vi "All-In-One_EIC-DIRC_DAQ_v2.vi"() -> ()   [LabVIEW 2024]
uses:
  C:/Users/hpDIRC/Desktop/eic_dirc_daq-LabVIEW_new/Thorlabs.MotionControl.Controls.dll
  Thorlabs.MotionControl.Controls.dll
  <vilib>/numeric/Random Number (Range) DBL.vi
  C:/Users/hpDIRC/Desktop/eic_dirc_daq-LabVIEW_new/Thorlabs.MotionControl.IntegratedStepperMotorsCLI.dll
  Thorlabs.MotionControl.IntegratedStepperMotorsCLI.dll
  C:/Users/hpDIRC/Desktop/eic_dirc_daq-LabVIEW_new/Thorlabs.MotionControl.Benchtop.StepperMotorCLI.dll
  Thorlabs.MotionControl.Benchtop.StepperMotorCLI.dll
  <instrlib>/Keithley 6517/Keithley 6517.lvlib
panel:
  in  "align-only":bool
  in  "run-BA":bool
  in  "run-IR":bool
  out "meter-mode":bool=TRUE
  in  "PDY start":dbl=105.8
  in  "PDX start":dbl=265.0
  out "run time (min)":dbl
  in  "align-only":bool
  out "alignment-counter":dbl=184.0 format="%#_13g"
  out "Optimized Location":dbl[](array[numeric])
  in  "Test Start Delay (s)":dbl=30.0
  out "Queue % Left":dbl format="%#_3g"
  out "next-state-cluster-const":T1={"next-state"="", "bypass-confirm"=FALSE, "PDX"=300.0, "PDY"=150.0, "BarX"=300.0, "BarY"=150.0, "BMA"=45.0, "PDA"=85.0, "bar-note"=0, "meas#"=0}
  in  "X start":dbl=262.0
  in  "X end":dbl=263.0
  in  "Y end":dbl=121.5 format="%#_13g"
  in  "X step size":dbl=0.2 format="%#_13g"
  in  "Y step size":dbl=0.2
  in  "Y start":dbl=120.5 format="%#_13g"
  in  "centered-diode-scan":bool
  out "keep-file":bool
  out "status":string
  out "queue-size":i32
  in  "save-loc":bool
  out "stored-pos":T2 caption="Location Stored"
  out "main-stage-refs":T3
  out "state-queue":T4(array[cluster])
  in  "PDA":dbl=184.0 format="%#_13g"
  in  "BMA":dbl=45.0 format="%#_13g"
  in  "BarY":dbl=30.0 format="%#_13g"
  in  "BarX":dbl=230.0 format="%#_13g"
  in  "PDY":dbl=124.0 format="%#_13g"
  in  "PDX":dbl=274.0 format="%#_13g"
  out "bypass-confirm":bool
  out "PD Values":cluster{"PD1":dbl, "PD2":dbl, "PD3":dbl}
  out "last-PD":dbl[](array[numeric])=[1.0, 1.0, 1.0]
  in  "move-bar":bool
  out "pd_angle":dbl
  out "brewster_angle":dbl
  out "meter-visa":refnum<visa-resource-name>
  out "loop-rate":u32
  out "meter-stat":bool caption="Log Status"
  out "file-stat":bool caption="Log Status"
  out "stage-stat":bool caption="Log Status"
  out "last-save-time":string caption="Time of Last Save:"
  out "pd_y_pos":dbl
  out "pd_x_pos":dbl
  out "bar_y_pos":dbl
  out "bar_x_pos":dbl
  in  "nSamples":dbl=50.0 caption="# Samples"
  out "Current Time:":string
  in  "save-data":bool
  in  "bar-note":u16(ring) items=["Pure Beam (PB)", "Internal Reflection (IR)", "Bulk Attenuation (BA)"]
  out "pd3_v":dbl caption="PD 3" format="%#.4g"
  out "pd2_v":dbl caption="PD 2" format="%#.4g"
  out "pd1_v":dbl caption="PD 1" format="%#.4g"
  out "meter-error":errorcluster
  out "log-error":errorcluster
  out "log-path":path caption="Path Data Will Save To:"
  out "start-msg":string
  out "stage-error":errorcluster
  in  "PD Angle":refnum<k24>(container)
  in  "Brewster":refnum<k24>(container)
  in  "PD Y":refnum<k24>(container)
  in  "PD X":refnum<k24>(container)
  in  "BAR Y":refnum<k24>(container)
  in  "stop":bool
  in  "BAR X":refnum<k24>(container)
  out "pd-plt":cluster{"[0]":dbl, "[1]":dbl, "[2]":dbl}(graph) caption="Measurement History"
  # "EXPERT DEBUGGING INFO"
  # "A"
  # "A"
  # "A"
  # "Work In Progress - please do not use"
  # "PD ONLY SCAN - CENTERED"
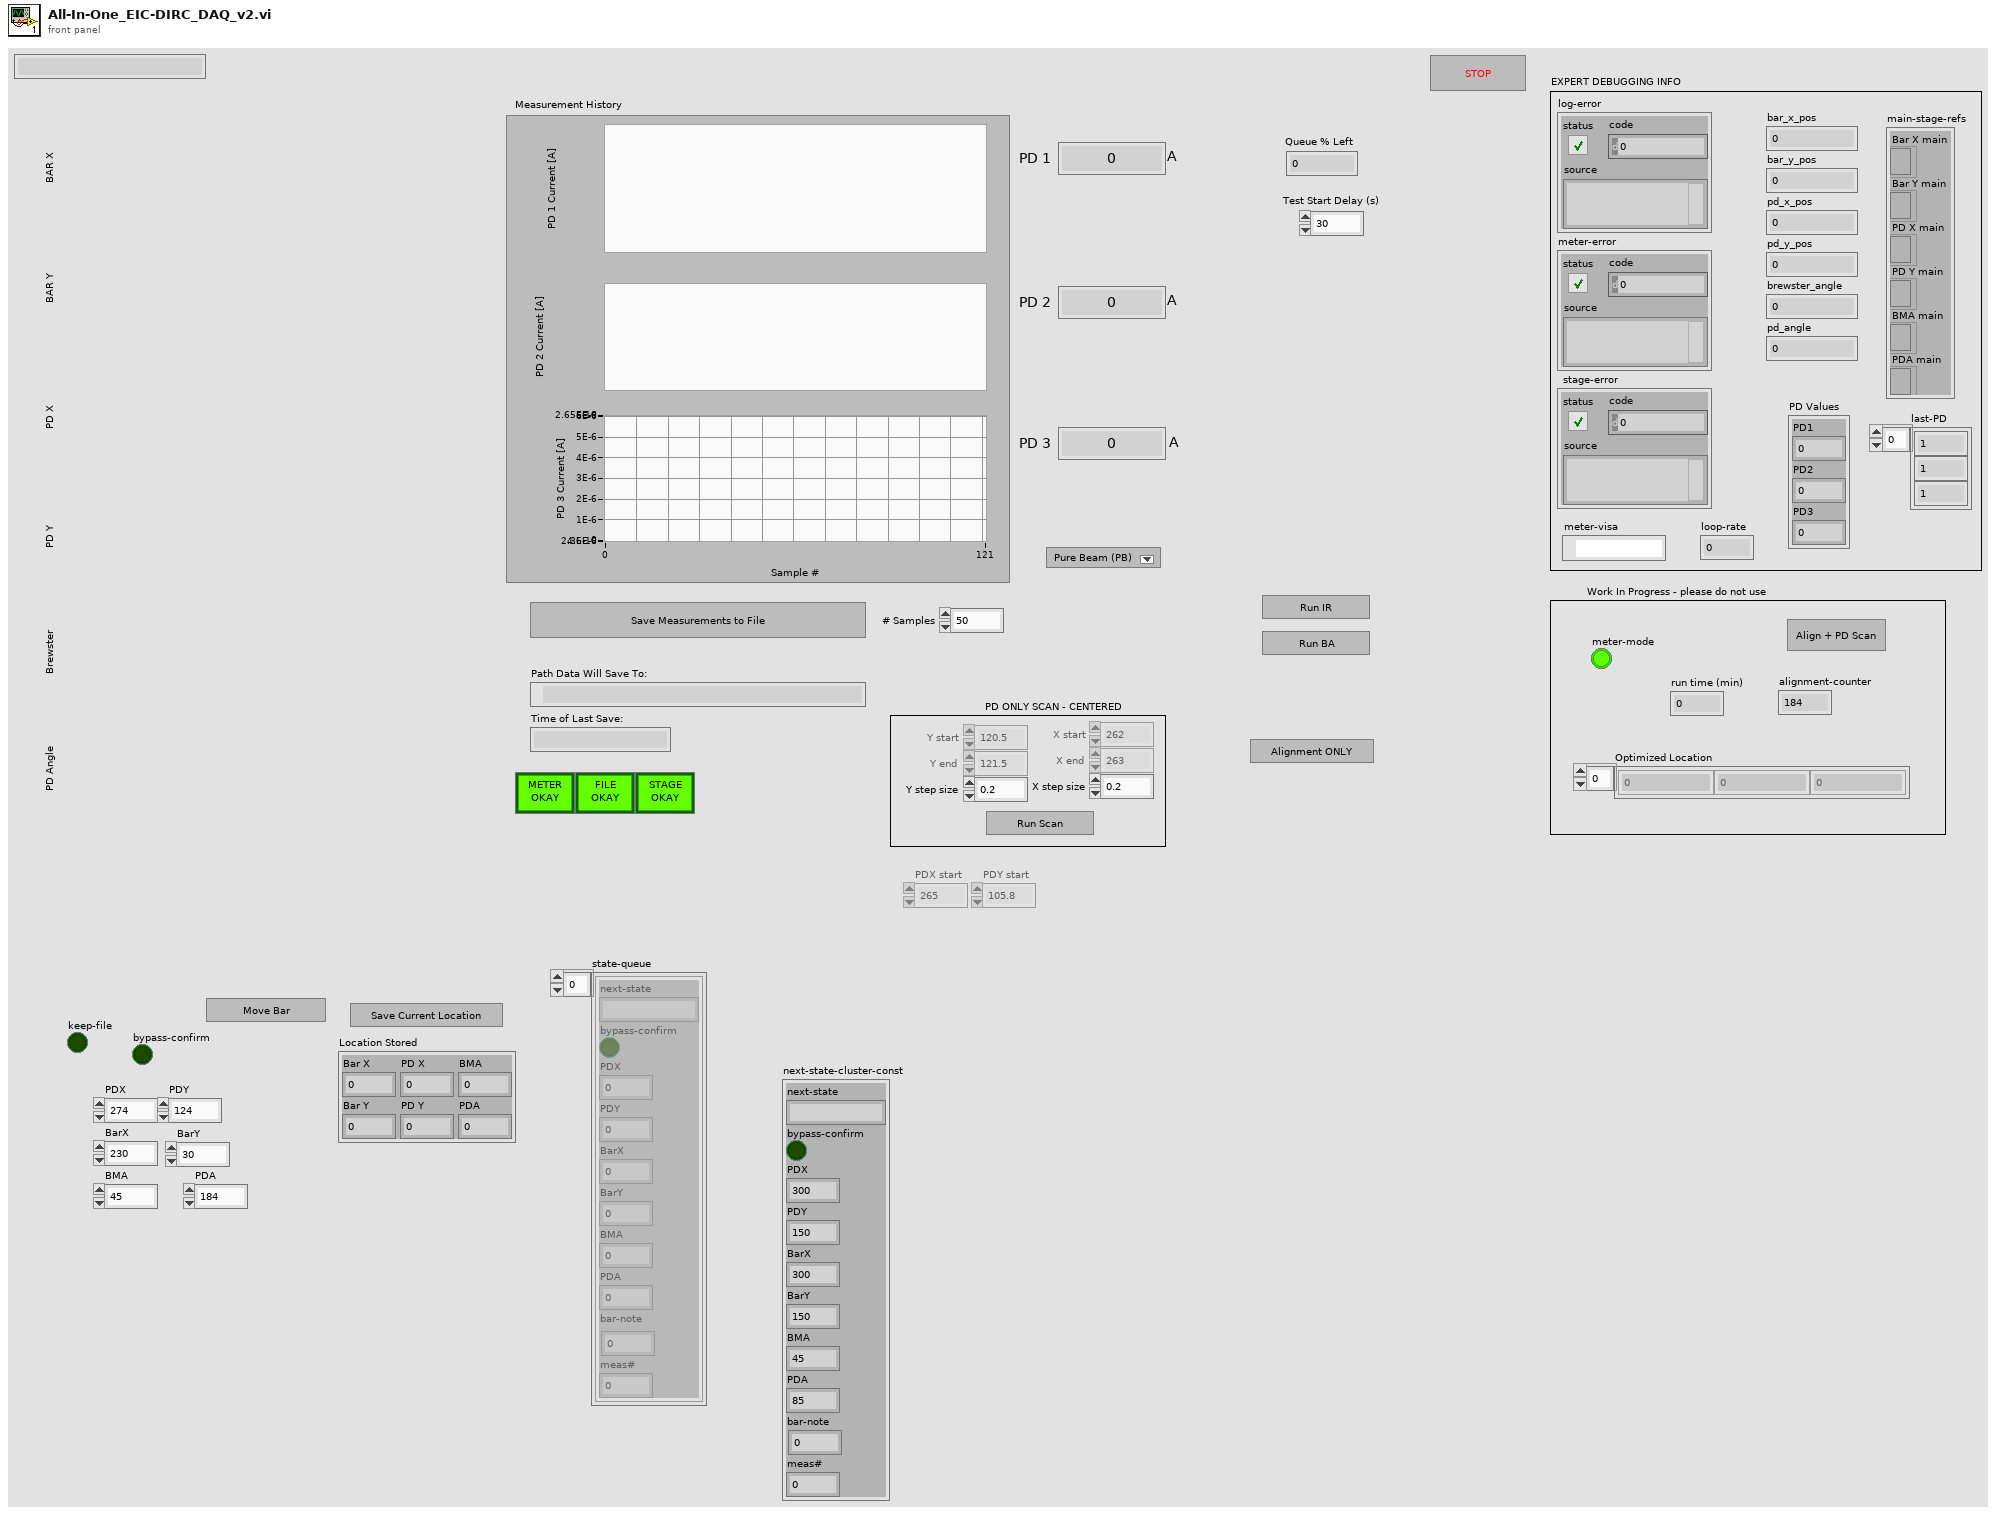
[diagram p1: front panel]
types:
  T1 = cluster{"next-state":string, "bypass-confirm":bool, "PDX":dbl, "PDY":dbl, "BarX":dbl, "BarY":dbl, "BMA":dbl, "PDA":dbl, "bar-note":u8, "meas#":u32}
  T2 = cluster{"Bar X":dbl, "Bar Y":dbl, "PD X":dbl, "PD Y":dbl, "BMA":dbl, "PDA":dbl}
  T3 = cluster{"Bar X main":refnum<k24>, "Bar Y main":refnum<k24>, "PD X main":refnum<k24>, "PD Y main":refnum<k24>, "BMA main":refnum<k24>, "PDA main":refnum<k24>}
  T4 = cluster{"next-state":string, "bypass-confirm":bool, "PDX":dbl, "PDY":dbl, "BarX":dbl, "BarY":dbl, "BMA":dbl, "PDA":dbl, "bar-note":u8, "meas#":u32}[]
  T5 = cluster{"Bar X":refnum<k24>, "Bar Y":refnum<k24>, "PD X":refnum<k24>, "PD Y":refnum<k24>, "Brewster":refnum<k24>, "PD Angle":refnum<k24>}
  T6 = enum16{"open", "replace", "create", "open or create", "replace or create", "replace or create with confirmation"}
  T7 = cluster{"alpha":dbl, "gamma":dbl, "rho":dbl, "sigma":dbl, "simplex L":dbl}
  T8 = cluster{"next-state":string, "mode-select":enum32{"IR", "Pure", "Bulk", "Bar Out", "stored-loc", "custom"}, "bypass-confirm":bool, "PDX":dbl, "PDY":dbl, "BarX":dbl, "BarY":dbl, "BMA":dbl, "PDA":dbl, "bar-note":bool}
  T9 = cluster{"error":bool, "code":i32, "source":string}
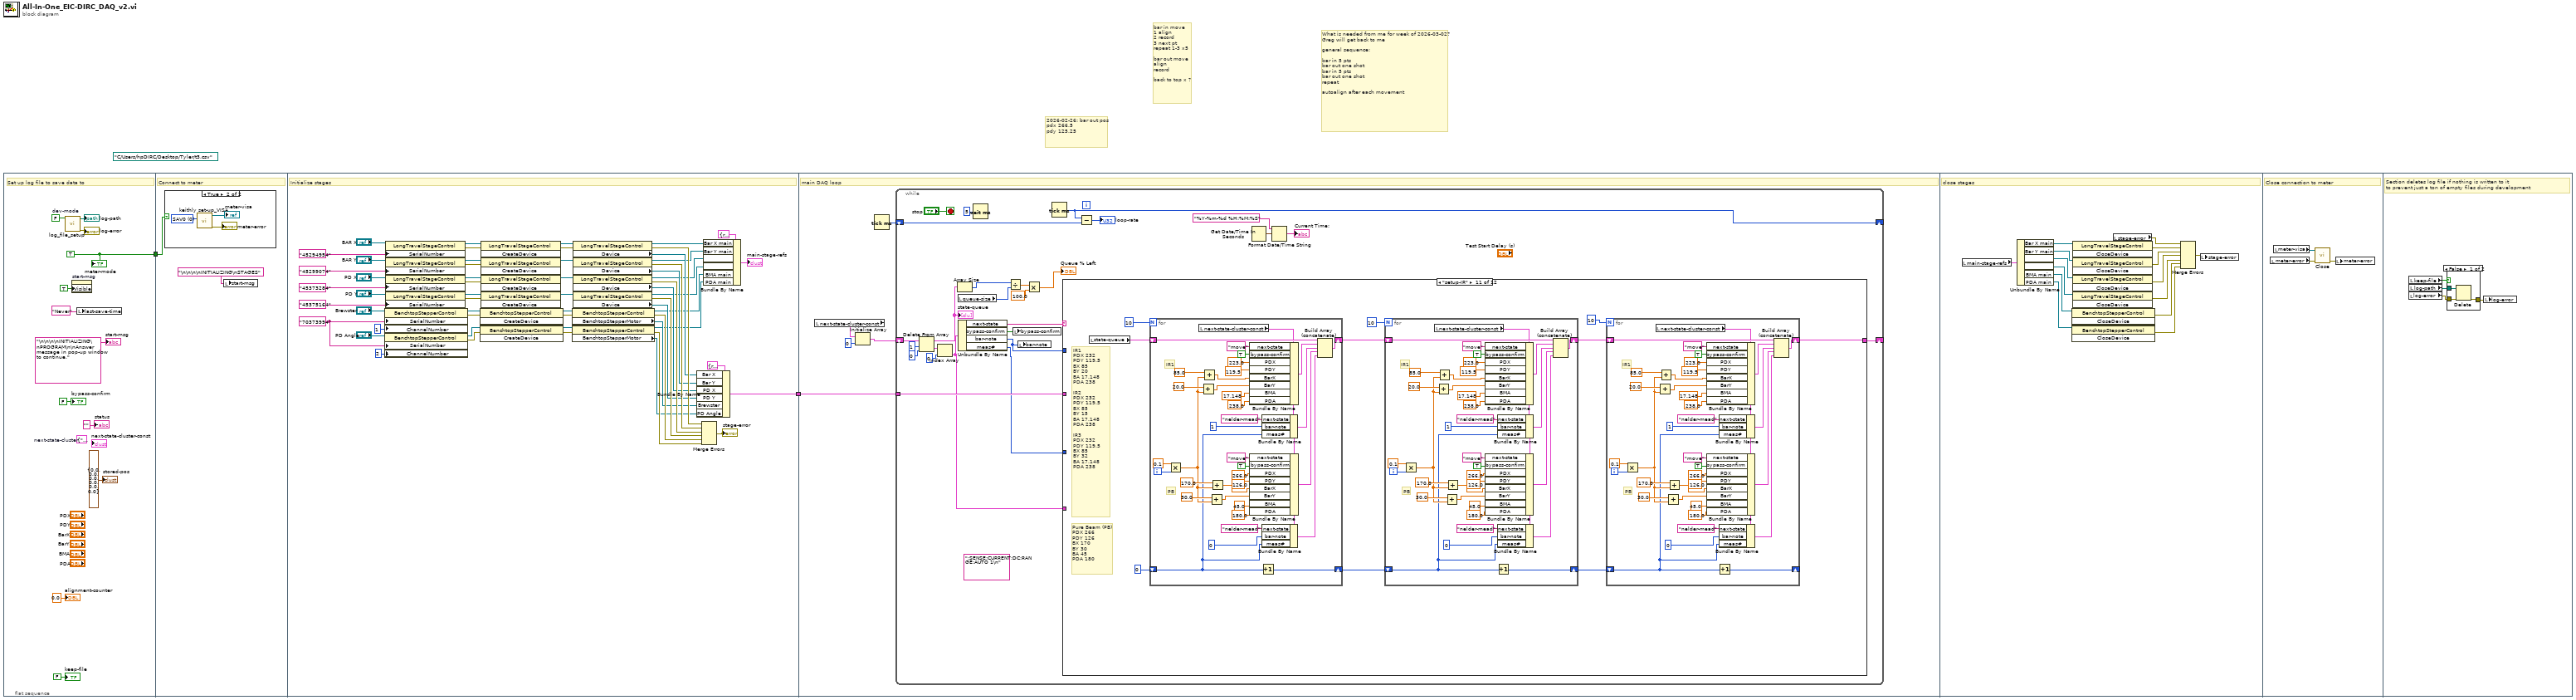
[diagram p0: block diagram]
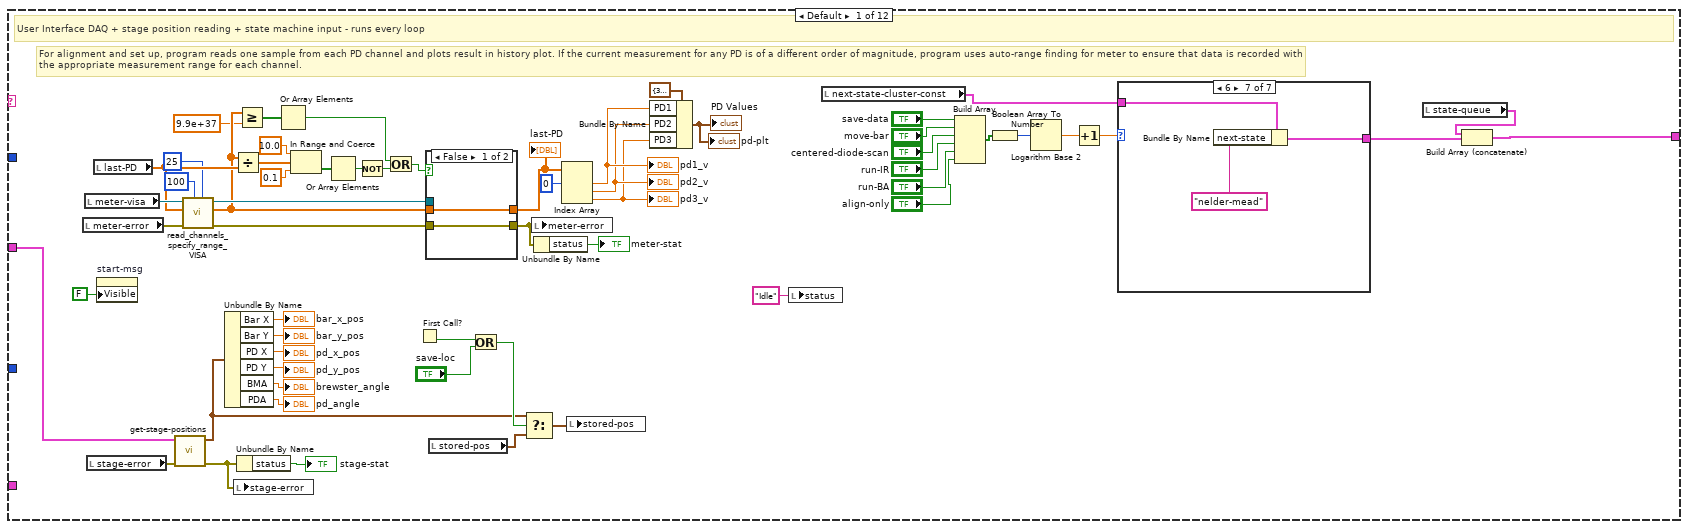
[diagram p3: hidden frame]
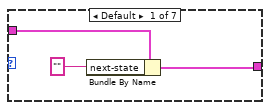
[diagram p4: hidden frame]
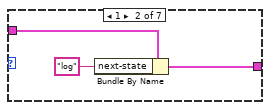
[diagram p5: hidden frame]
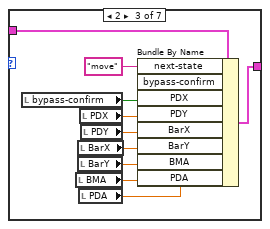
[diagram p6: hidden frame]
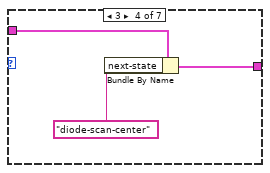
[diagram p7: hidden frame]
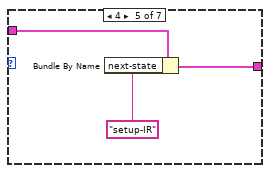
[diagram p8: hidden frame]
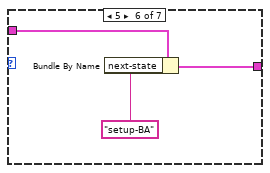
[diagram p9: hidden frame]
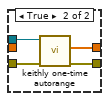
[diagram p10: hidden frame]
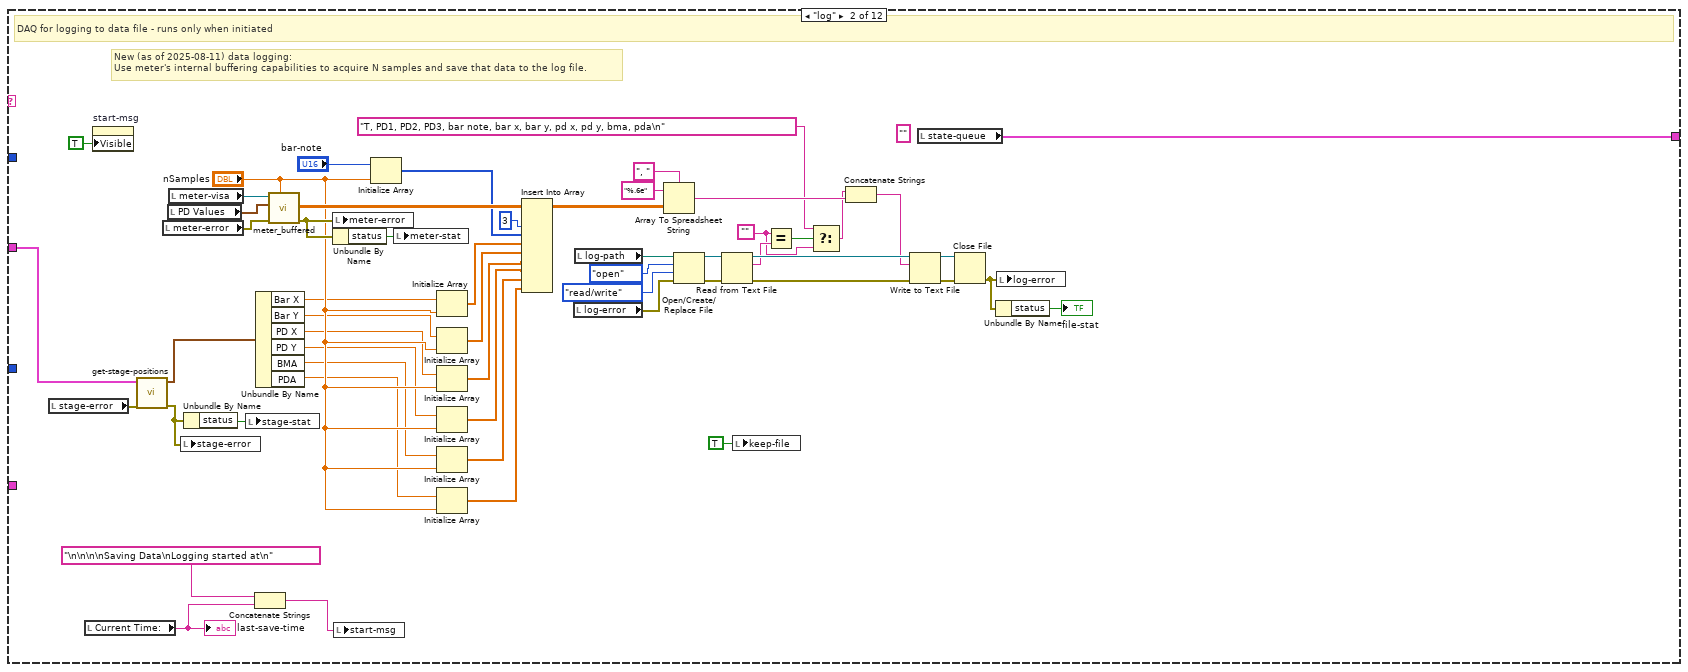
[diagram p11: hidden frame]
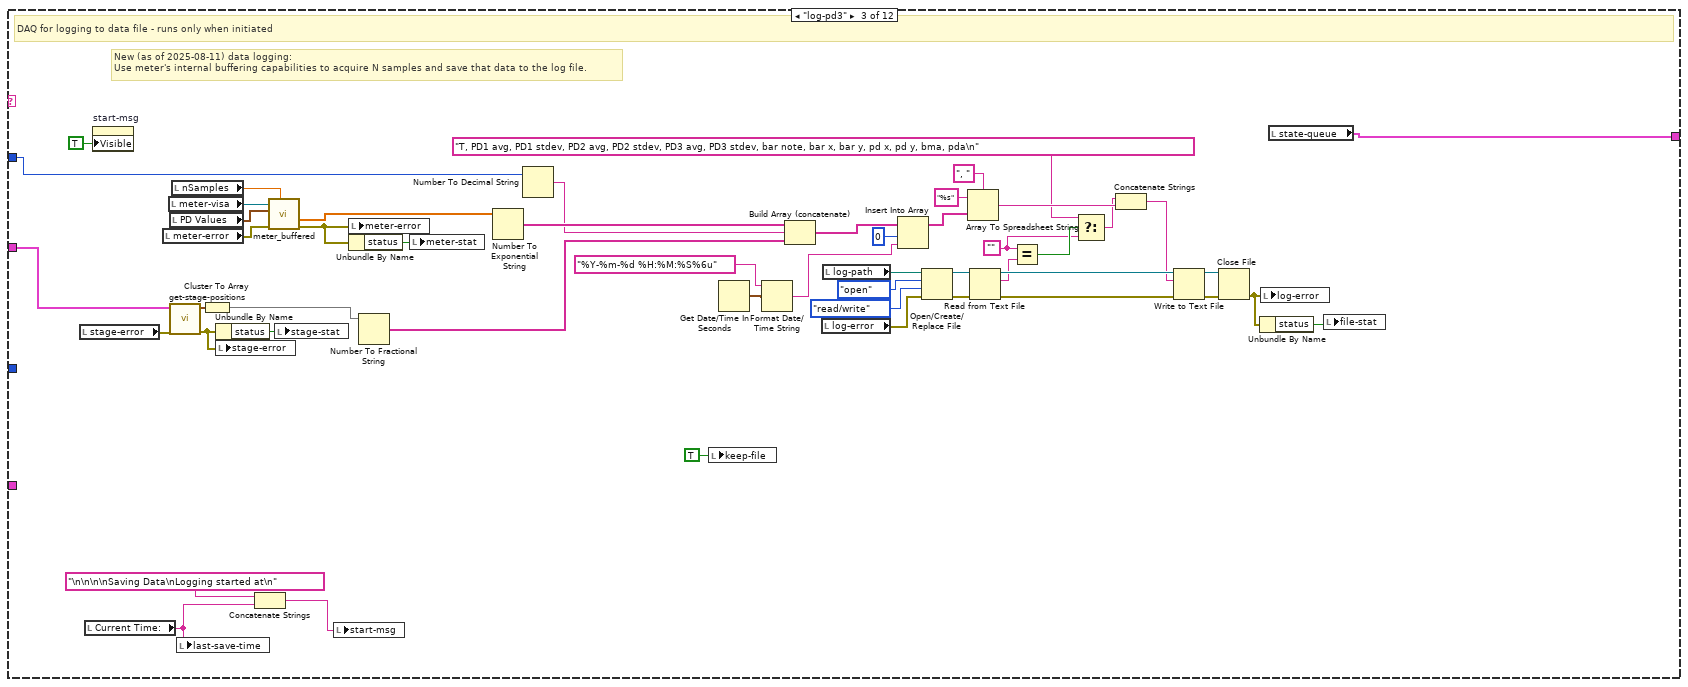
[diagram p12: hidden frame]
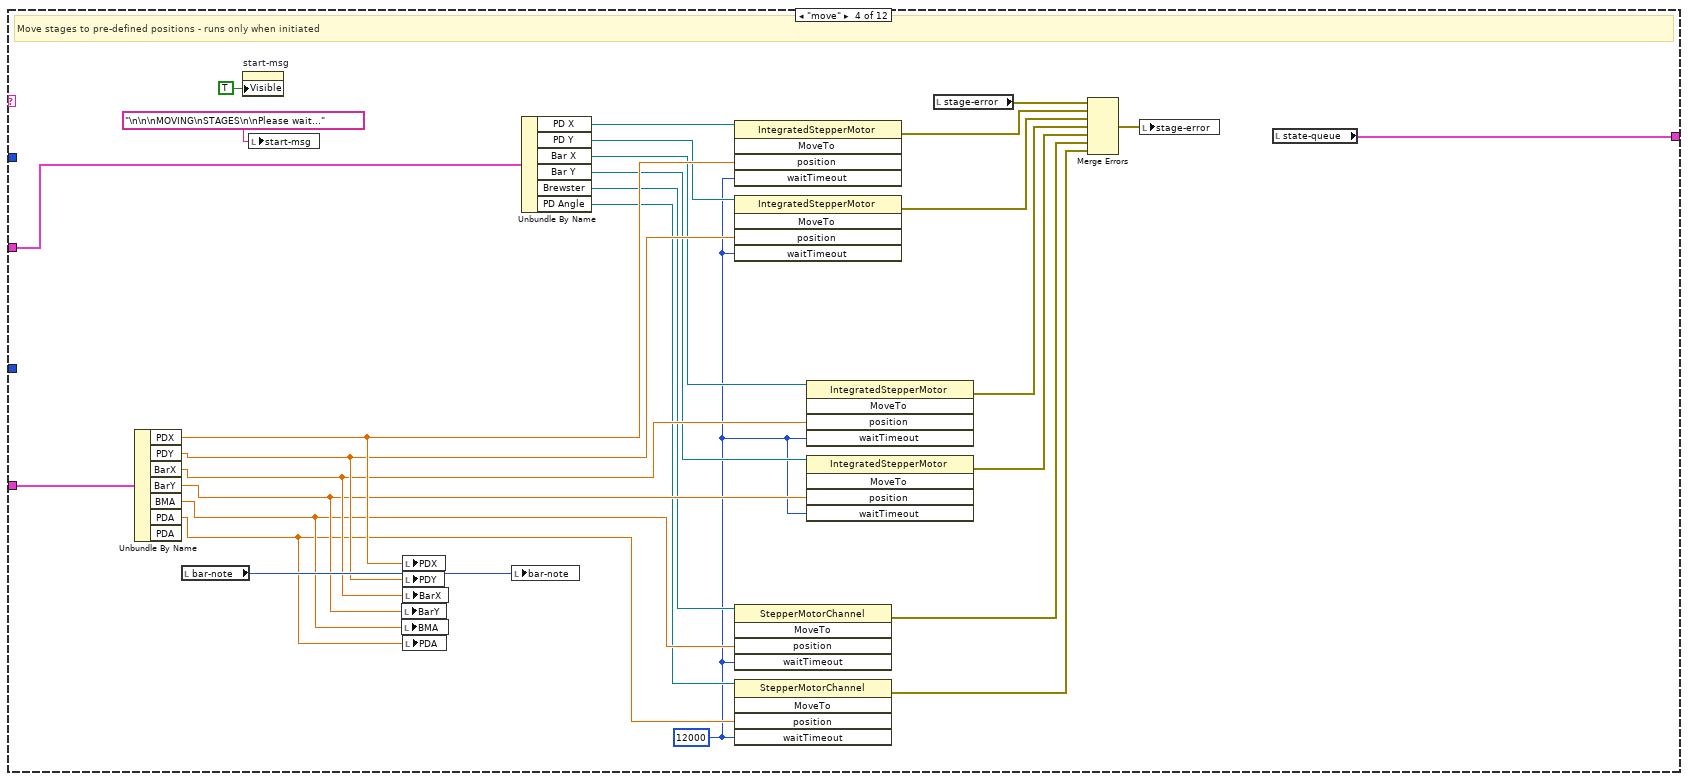
[diagram p13: hidden frame]
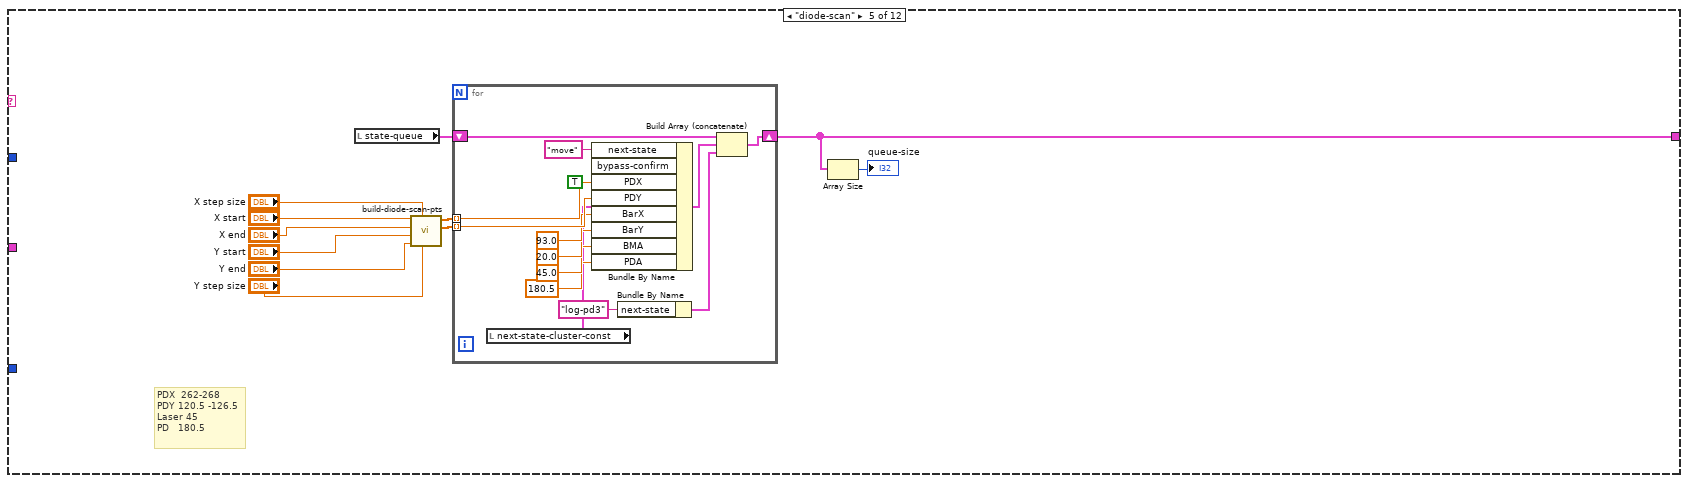
[diagram p14: hidden frame]
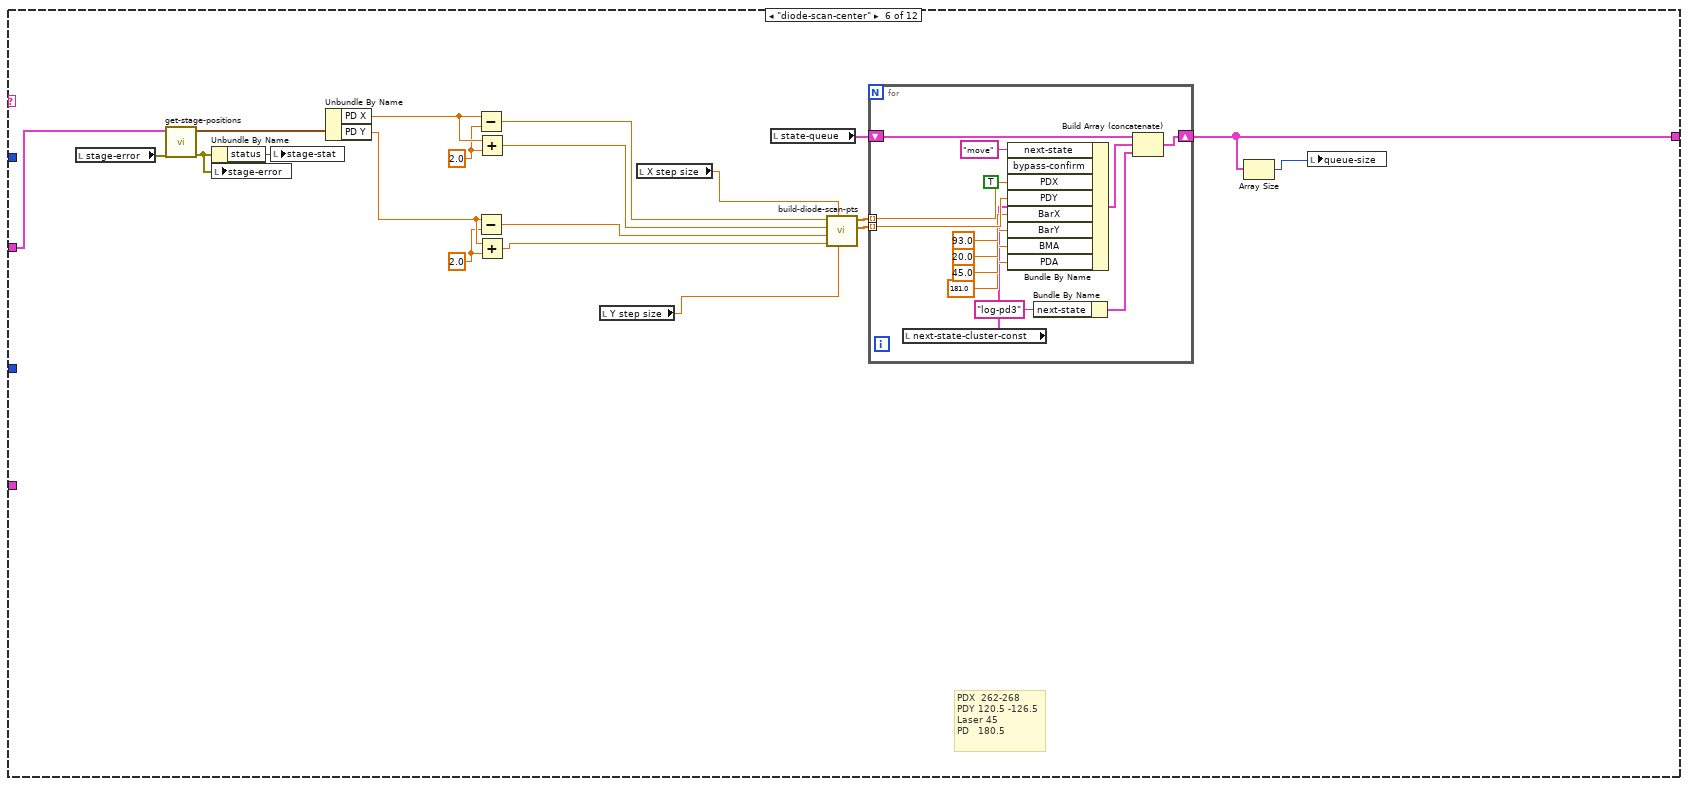
[diagram p15: hidden frame]
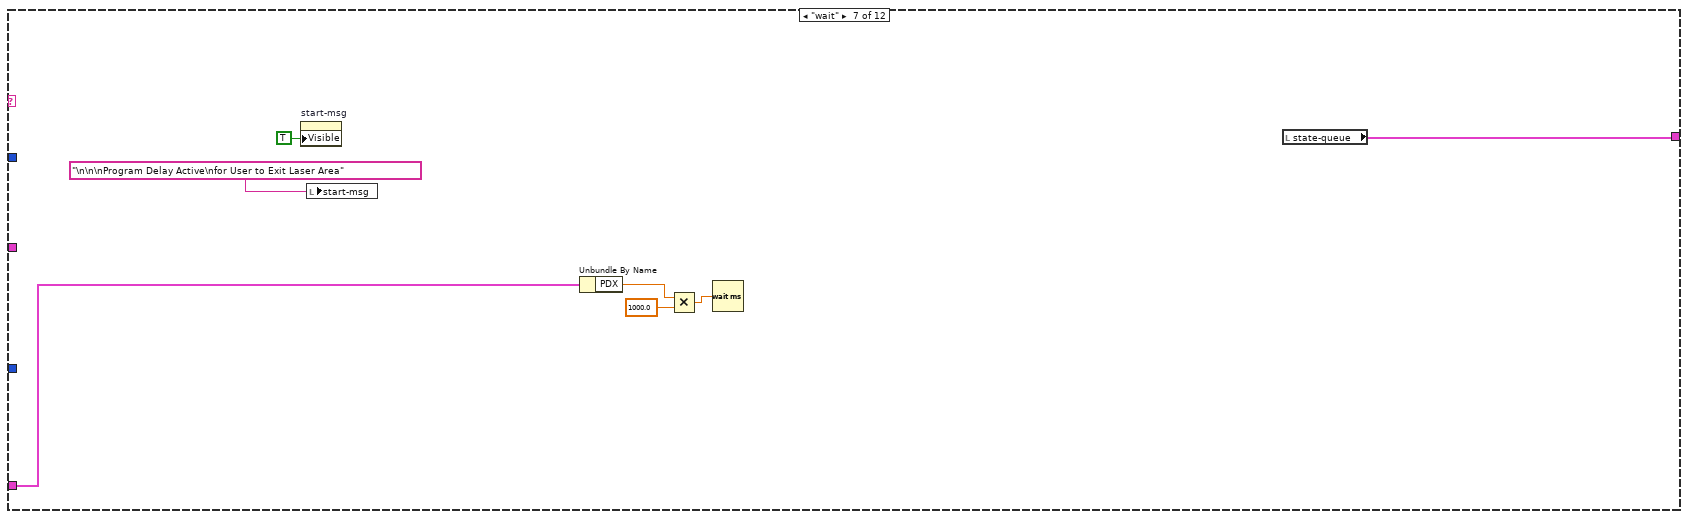
[diagram p16: hidden frame]
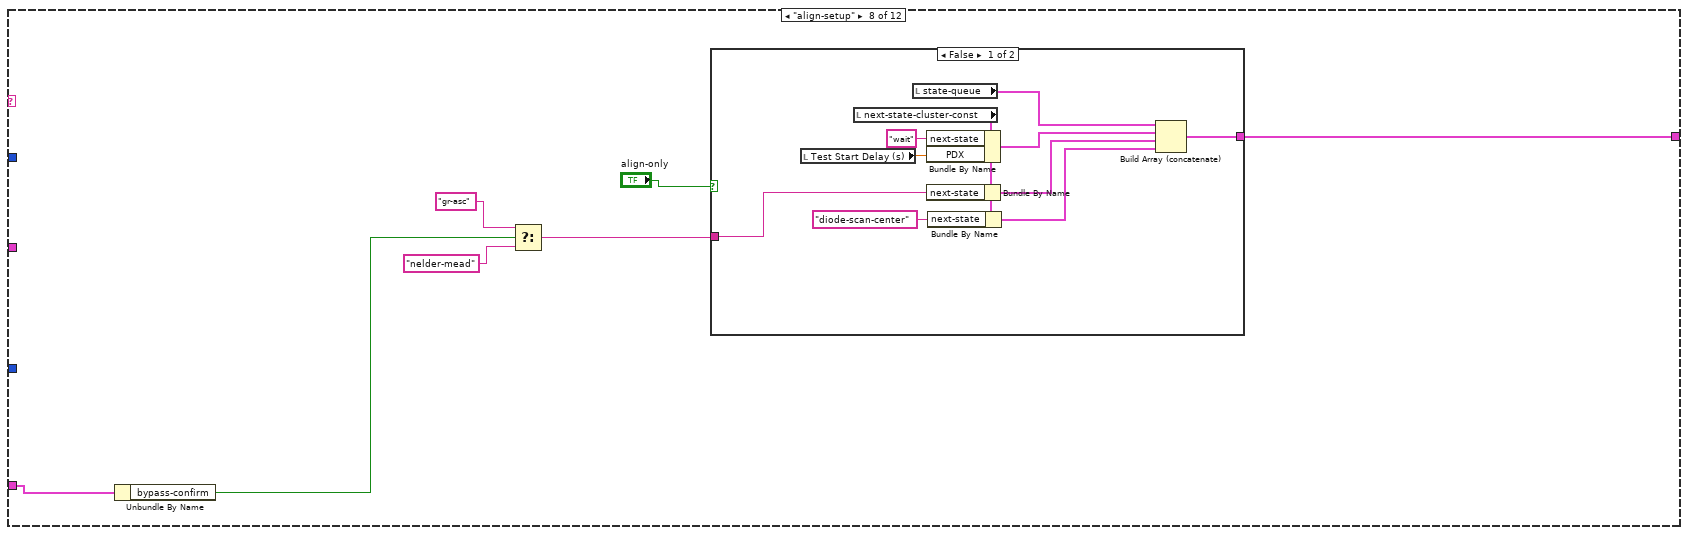
[diagram p17: hidden frame]
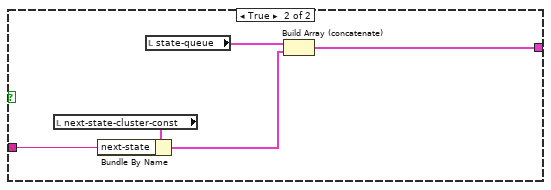
[diagram p18: hidden frame]
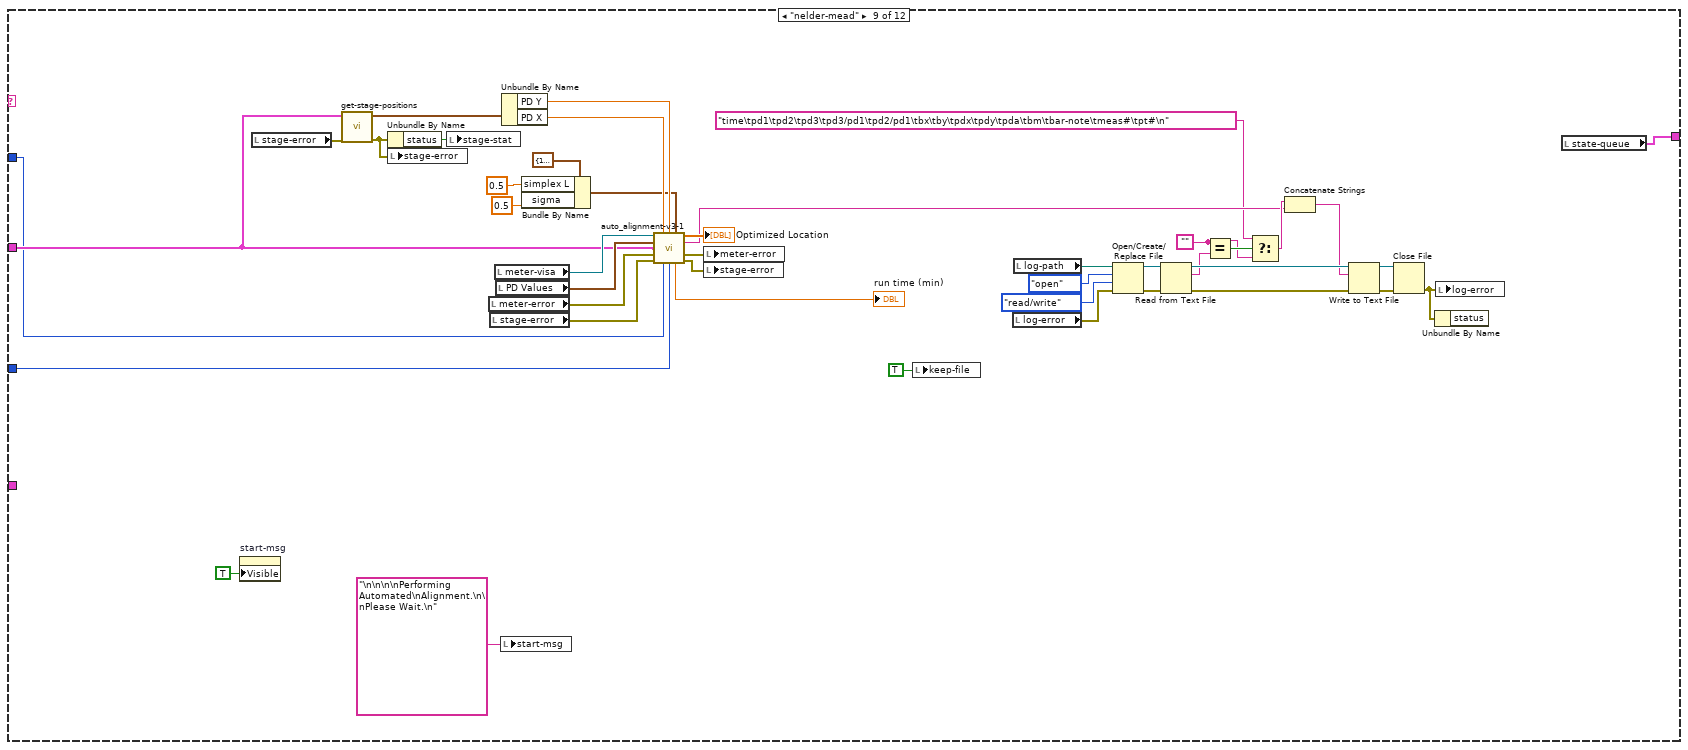
[diagram p19: hidden frame]
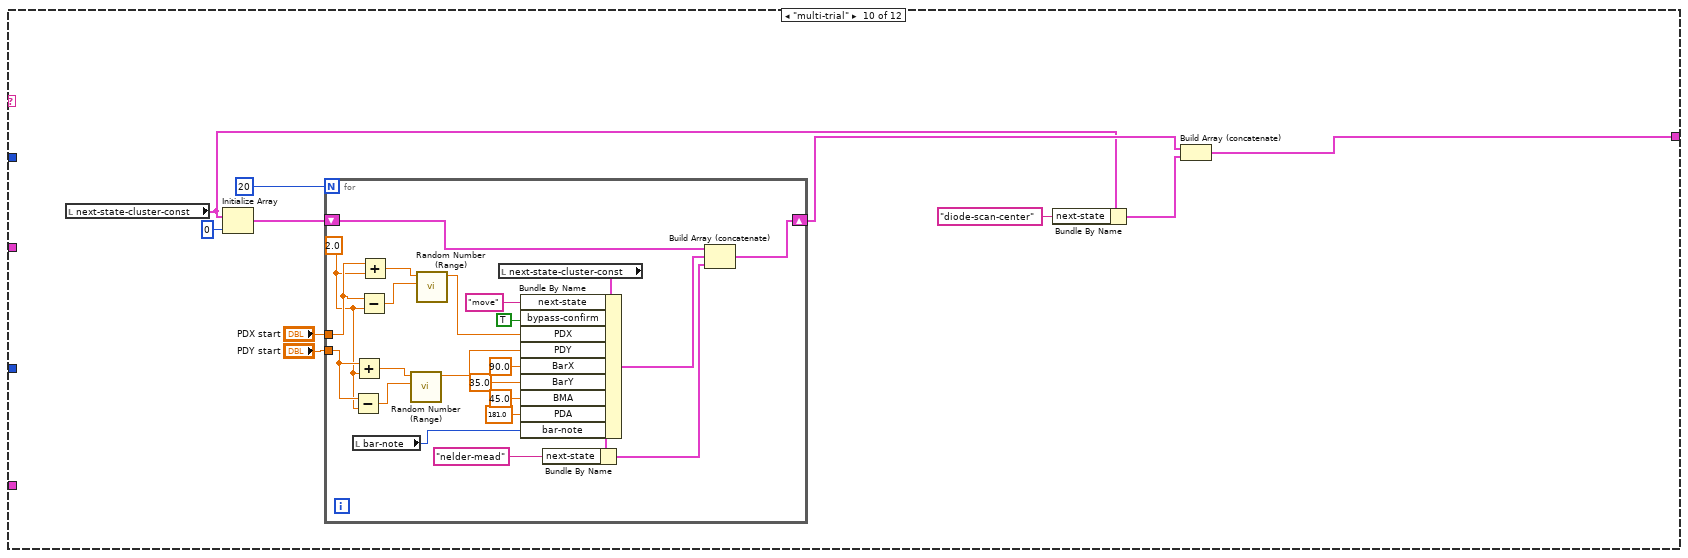
[diagram p20: hidden frame]
diagram:
  (unwired) path "C:/Users/hpDIRC/Desktop/Tyler/t3.csv" ("log-path")
  # "2026-02-26: bar out pos\npdx 266.5\npdy 125.25"
  # "bar in move\n1 align\n2 record\n3 next pt\nrepeat 1-3 x5\n\nbar out move\nalign\nrecord\n\nback to top x ?"
  # "What is needed from me for week of 2026-03-02?\nGreg will get back to me\n\ngeneral sequence:\n\nbar in 5 pts \nbar out one shot\nbar in 5 pts\nbar out one shot\nrepeat\n\nautoalign after each movement"
  n1 = flat-sequence {
    tunnel: [w3] -> w1
    tunnel: w1 -> [w15]
    tunnel: [w28] -> w2
    tunnel: w2 -> [w80]
    frame #0 {
      w3 = TRUE
      (unwired) T8 {"next-state"="", "mode-select"=enum."IR", "bypass-confirm"=FALSE, "PDX"=300.0, "PDY"=150.0, "BarX"=300.0, "BarY"=150.0, "BMA"=45.0, "PDA"=85.0, "bar-note"=FALSE}  # next-state-cluster
      w14 = FALSE  # dev-mode
      # "Set up log file to save data to"
      n2 = call "log_file_setup.vi"("dev-mode"=w14) -> ("error out"=→"log-error":errorcluster, "appended path"=→"log-path":path)  [unwired: 8 in, 1 out]
      n3 = property on="start-msg" class="Str"("Visible"=TRUE) -> ()  [unwired: 2 in, 2 out]
      n4 = local write "last-save-time"("Never" ("date/time string")) -> ()
      "start-msg" <- "\n\n\n\nINITIALIZING\nPROGRAM\n\nAnswer message in pop-up window to continue." ("String")
      "bypass-confirm" <- FALSE
      "stored-pos" <- T2 {"Bar X"=0.0, "Bar Y"=0.0, "PD X"=0.0, "PD Y"=0.0, "BMA"=0.0, "PDA"=0.0} ("stage-pos")
      "status" <- "" ("status")
      "keep-file" <- FALSE
      "alignment-counter" <- 0.0 ("alignment-counter")
      "meter-mode" <- w3
    }
    frame #1 {
      # "Connect to meter"
      n5 = case shown="True" w15 {
        frame False {
        }
        frame True {
          w17 = i16 0 items=["SAV0", "SAV1", "SAV2", "SAV3", "SAV4", "SAV5", "SAV6", "SAV7", "SAV8", "SAV9", "RST", "Preset"] ("ConfigOpt")
          n6 = call "keithly set-up_VISA.vi"("ConfigOpt"=w17) -> ("error out"=→"meter-error":errorcluster, "meter-VISA"=→"meter-visa":refnum<visa-resource-name>)  [unwired: 9 in]
        }
      }
      n7 = local write "start-msg"("\n\n\n\nINITIALIZING\nSTAGES" ("String")) -> ()
    }
    frame #2 {
      w35 = "70373994" ("SerialNumber")
      # "Initialize stages"
      n8 = property class="BenchtopStepperControl"(reference="Brewster", "SerialNumber"=w35, "ChannelNumber"=1) -> (reference out=w61:refnum<k24>, error out=w62:errorcluster)  [unwired: 1 in]
      n9 = property class="BenchtopStepperControl"(reference="PD Angle", "SerialNumber"=w35, "ChannelNumber"=2) -> (reference out=w60:refnum<k24>, error out=w63:errorcluster)  [unwired: 1 in]
      n10 = property class="LongTravelStageControl"(reference="BAR X", "SerialNumber"="45294954") -> (reference out=w38:refnum<k24>, error out=w45:errorcluster)  [unwired: 1 in]
      n11 = property class="LongTravelStageControl"(reference="BAR Y", "SerialNumber"="45299074") -> (reference out=w39:refnum<k24>, error out=w46:errorcluster)  [unwired: 1 in]
      n12 = property class="LongTravelStageControl"(reference="PD X", "SerialNumber"="45373284") -> (reference out=w42:refnum<k24>, error out=w47:errorcluster)  [unwired: 1 in]
      n13 = property class="LongTravelStageControl"(reference="PD Y", "SerialNumber"="45375164") -> (reference out=w43:refnum<k24>, error out=w48:errorcluster)  [unwired: 1 in]
      n14 = invoke class="BenchtopStepperControl" method="CreateDevice"(reference=w61, error in=w62) -> (reference out=w58:refnum<k24>, error out=w56:errorcluster)  [unwired: 1 in, 1 out]
      n15 = invoke class="BenchtopStepperControl" method="CreateDevice"(reference=w60, error in=w63) -> (reference out=w57:refnum<k24>, error out=w59:errorcluster)  [unwired: 1 in, 1 out]
      n16 = invoke class="LongTravelStageControl" method="CreateDevice"(reference=w38, error in=w45) -> (reference out=w51:refnum<k24>, error out=w55:errorcluster)  [unwired: 1 in, 1 out]
      n17 = invoke class="LongTravelStageControl" method="CreateDevice"(reference=w39, error in=w46) -> (reference out=w52:refnum<k24>)  [unwired: 1 in, 2 out]
      n18 = invoke class="LongTravelStageControl" method="CreateDevice"(reference=w42, error in=w47) -> (reference out=w53:refnum<k24>)  [unwired: 1 in, 2 out]
      n19 = invoke class="LongTravelStageControl" method="CreateDevice"(reference=w43, error in=w48) -> (reference out=w54:refnum<k24>)  [unwired: 1 in, 2 out]
      n20 = property class="BenchtopStepperControl"(reference=w58, error in=w56) -> (reference out=w22:refnum<k24>, error out=w73:errorcluster, "BenchtopStepperMotor"=w68:refnum<k24>)
      n21 = property class="BenchtopStepperControl"(reference=w57, error in=w59) -> (reference out=w21:refnum<k24>, error out=w74:errorcluster, "BenchtopStepperMotor"=w69:refnum<k24>)
      n22 = property class="LongTravelStageControl"(reference=w51, error in=w55) -> (reference out=w26:refnum<k24>, error out=w75:errorcluster, "Device"=w64:refnum<k24>)
      n23 = property class="LongTravelStageControl"(reference=w52) -> (reference out=w25:refnum<k24>, error out=w70:errorcluster, "Device"=w65:refnum<k24>)  [unwired: 1 in]
      n24 = property class="LongTravelStageControl"(reference=w53) -> (reference out=w24:refnum<k24>, error out=w71:errorcluster, "Device"=w66:refnum<k24>)  [unwired: 1 in]
      n25 = property class="LongTravelStageControl"(reference=w54) -> (reference out=w23:refnum<k24>, error out=w72:errorcluster, "Device"=w67:refnum<k24>)  [unwired: 1 in]
      n26 = Bundle By Name(cluster=T5 {"Bar X"=refnum, "Bar Y"=refnum, "PD X"=refnum, "PD Y"=refnum, "Brewster"=refnum, "PD Angle"=refnum}, "Bar X"=w64, "Bar Y"=w65, "PD X"=w66, "PD Y"=w67, "Brewster"=w68, "PD Angle"=w69) -> (w28:T5)
      n27 = Merge Errors(w75, w70, w71, w72, w73, w74) -> (→"stage-error":errorcluster)
      n28 = Bundle By Name(cluster=T3 {"Bar X main"=refnum, "Bar Y main"=refnum, "PD X main"=refnum, "PD Y main"=refnum, "BMA main"=refnum, "PDA main"=refnum}, "Bar X main"=w26, "Bar Y main"=w25, "PD X main"=w24, "PD Y main"=w23, "BMA main"=w22, "PDA main"=w21) -> (→"main-stage-refs":T3)
    }
    frame #3 {
      # "main DAQ loop"
      n29 = local read "next-state-cluster-const"() -> (w77:T1)
      n30 = Initialize Array(w77, 0 ("dimension size")) -> (w79:T4)
      n31 = Tick Count (ms)() -> (millisecond timer value=w81:u32)
      n32 = while {
        shift-right: [w106] -> _
        shift-left: w81 -> [w105]
        tunnel: w80 -> [w103]
        shift-right: [w91] -> _
        shift-left: w79 -> [w93]
        stop <- "stop" stop-if-true
        (unwired) ":SENSE:CURRENT:DC:RANGE:AUTO 1\n"
        n33 = Delete From Array(array=w93, length=1, index=0) -> (deleted portion=w92:T4, array with subset deleted=w89:T4)
        "state-queue" <- w89
        n34 = Index Array(array=w92, index=0) -> (element=w90:T1)
        n35 = Array Size(array=w89) -> (size(s)=w84:i32)
        n36 = local read "queue-size"() -> (w88:i32)
        n37 = Unbundle By Name(w90) -> ("next-state"=w95:string, "bypass-confirm"=w94:bool, "bar-note"=w83:u8, "meas#"=w82:u32)
        n38 = Wait (ms)(milliseconds to wait=u32 5) -> ()  [unwired: 1 out]
        n39 = Divide(x=w84, y=w88) -> (x/y=w87:dbl)
        n40 = local write "bypass-confirm"(w94) -> ()
        n41 = local write "bar-note"(w83) -> ()
        n42 = Multiply(x=w87, y=100.0) -> (x*y=→"Queue % Left":dbl)
        n43 = Tick Count (ms)() -> (millisecond timer value=w106:u32)
        n44 = case shown="\"setup-IR\"" w95 {
          tunnel: w103 -> [w158 w219 w284 w331 _ w366 _ _ w442 _ _ _]
          tunnel: [w130 w230 w289 w330 w340 w374 w394 w400 w463 w466 w496 w614] -> w91
          tunnel: w90 -> [_ _ _ w327 _ _ w395 w405 _ _ _ _]
          tunnel: w83 -> [_ _ w267 _ _ _ _ _ w441 _ _ _]
          tunnel: w82 -> [_ _ _ _ _ _ _ _ w440 _ _ _]
          frame Default {
            # "For alignment and set up, program reads one sample from each PD channel and plots result in history plot. If the current measurement for any PD is of a different order of magnitude, program uses auto-range finding for meter to ensure that data is recorded with the appropriate measurement range for each channel."
            # "User Interface DAQ + stage position reading + state machine input - runs every loop"
            n45 = local read "meter-error"() -> (w155:errorcluster)
            n46 = local read "meter-visa"() -> (w156:refnum<visa-resource-name>)
            n47 = local read "stage-error"() -> (w157:errorcluster)
            n48 = local read "last-PD"() -> (w146:dbl[])
            n49 = property on="start-msg" class="Str"("Visible"=FALSE) -> ()  [unwired: 2 in, 2 out]
            n50 = call "get-stage-positions.vi"("error in (no error)"=w157, "Cluster"=w158) -> ("error out"=w143:errorcluster, "stage positions"=w116:T2)  [unwired: 8 in]
            n51 = call "read_channels_specify_range_VISA.vi"("postDAQ  wait ms"=u32 25, "preDAQ  wait ms"=u32 100, "error in"=w155, "range"=w146, "VISA resource in"=w156) -> ("error out"=w148:T9, "data"=w136:dbl[], "VISA resource out"=w147:refnum<visa-resource-name>)  [unwired: 4 in]
            n52 = Unbundle By Name(w116) -> ("Bar X"=→"bar_x_pos":dbl, "Bar Y"=→"bar_y_pos":dbl, "PD X"=→"pd_x_pos":dbl, "PD Y"=→"pd_y_pos":dbl, "BMA"=→"brewster_angle":dbl, "PDA"=→"pd_angle":dbl)
            n53 = Divide(x=w136, y=w146) -> (x/y=w151:dbl[])
            n54 = local write "stage-error"(w143) -> ()
            n55 = Greater Or Equal?(x=w136, y=9.9e+37) -> (x >= y?=w134:bool[])
            n56 = Unbundle By Name(w143) -> ("status"=→"stage-stat":bool)
            n57 = Or Array Elements(Boolean array=w134) -> (logical OR=w133:bool)
            n58 = In Range and Coerce(upper limit=10.0, x=w151, lower limit=0.1) -> (In Range?=w149:bool[])  [unwired: 1 out]
            n59 = Or Array Elements(Boolean array=w149) -> (logical OR=w150:bool)
            n60 = Not(x=w150) -> (.not. x?=w138:bool)
            n61 = Or(x=w133, y=w138) -> (x .or. y?=w137:bool)
            n62 = First Call?() -> (First Call?: T/F=w126:bool)
            n63 = case shown="False" w137 {
              tunnel: w148 -> [w196 w200]
              tunnel: [w196 w199] -> w164
              tunnel: [w195 w198] -> w159
              tunnel: w136 -> [w195 _]
              tunnel: w147 -> [_ w197]
              frame False {
              }
              frame True {
                n64 = call "keithly one-time autorange.vi"("error in"=w200, "VISA in"=w197) -> ("error out"=w199:errorcluster, "data"=w198:dbl[])  [unwired: 7 in, 1 out]
              }
            }
            "last-PD" <- w159
            n65 = local read "stored-pos"() -> (w127:T2)
            n66 = Or(x=w126, y="save-loc") -> (x .or. y?=w124:bool)
            n67 = Select(t=w116, s=w124, f=w127) -> (s? t:f=w128:T2)
            n68 = local write "meter-error"(w164) -> ()
            n69 = Unbundle By Name(w164) -> ("status"=→"meter-stat":bool)
            n70 = Index Array(array=w159, index #1=0 ("index")) -> (element #1=w162:dbl, element #2=w161:dbl, element #3=w160:dbl)  [unwired: 2 in]
            "pd3_v" <- w160
            "pd2_v" <- w161
            "pd1_v" <- w162
            n71 = local write "stored-pos"(w128) -> ()
            n72 = Bundle By Name(cluster=cluster{"PD1":dbl, "PD2":dbl, "PD3":dbl} {"PD1"=3e-05, "PD2"=3e-05, "PD3"=3e-05} ("PD ranges"), "PD1"=w162, "PD2"=w161, "PD3"=w160) -> (→"pd-plt" →"PD Values":cluster{"PD1":dbl, "PD2":dbl, "PD3":dbl})
            n73 = local write "status"("Idle" ("status")) -> ()
            n74 = local read "next-state-cluster-const"() -> (w114:T1)
            n75 = Build Array("save-data", "move-bar", "centered-diode-scan", "run-IR", "run-BA", "align-only") -> (w140:bool[])
            n76 = Boolean Array To Number(Boolean array=w140) -> (number=w111:u32)
            n77 = Logarithm Base 2(1:w111) -> (0:w113:dbl)
            n78 = Increment(x=w113) -> (x+1=w112:dbl)
            n79 = case shown="6" w112 {
              tunnel: w114 -> [w169 w172 w182 w185 w188 w191 w194]
              tunnel: [w167 w170 w180 w183 w186 w189 w192] -> w129
              frame Default {
                n80 = Bundle By Name(cluster=w169, "next-state"="") -> (w167:T1)
              }
              frame 1 {
                n81 = Bundle By Name(cluster=w172, "next-state"="log") -> (w170:T1)
              }
              frame 2 {
                n82 = local read "bypass-confirm"() -> (w173:bool)
                n83 = local read "BMA"() -> (w178:dbl)
                n84 = local read "BarX"() -> (w176:dbl)
                n85 = local read "BarY"() -> (w177:dbl)
                n86 = local read "PDA"() -> (w179:dbl)
                n87 = local read "PDX"() -> (w174:dbl)
                n88 = local read "PDY"() -> (w175:dbl)
                n89 = Bundle By Name(cluster=w182, "next-state"="move", "bypass-confirm"=w173, "PDX"=w174, "PDY"=w175, "BarX"=w176, "BarY"=w177, "BMA"=w178, "PDA"=w179) -> (w180:T1)
              }
              frame 3 {
                n90 = Bundle By Name(cluster=w185, "next-state"="diode-scan-center") -> (w183:T1)
              }
              frame 4 {
                n91 = Bundle By Name(cluster=w188, "next-state"="setup-IR") -> (w186:T1)
              }
              frame 5 {
                n92 = Bundle By Name(cluster=w191, "next-state"="setup-BA") -> (w189:T1)
              }
              frame 6 {
                n93 = Bundle By Name(cluster=w194, "next-state"="nelder-mead") -> (w192:T1)
              }
            }
            n94 = local read "state-queue"() -> (w131:T4)
            n95 = Build Array (concatenate)(w131, w129) -> (w130:T4)
          }
          frame "log" {
            w205 = ""
            (unwired) ""
            # "New (as of 2025-08-11) data logging:\nUse meter's internal buffering capabilities to acquire N samples and save that data to the log file."
            # "DAQ for logging to data file - runs only when initiated"
            n96 = local read "stage-error"() -> (w218:errorcluster)
            n97 = local read "Current Time:"() -> (w228:string)
            "last-save-time" <- w228
            n98 = property on="start-msg" class="Str"("Visible"=TRUE) -> ()  [unwired: 2 in, 2 out]
            n99 = call "get-stage-positions.vi"("error in (no error)"=w218, "Cluster"=w219) -> ("error out"=w217:errorcluster, "stage positions"=w215:T2)  [unwired: 8 in]
            n100 = local read "meter-error"() -> (w254:errorcluster)
            n101 = local read "PD Values"() -> (w233:cluster{"PD1":dbl, "PD2":dbl, "PD3":dbl})
            n102 = local read "meter-visa"() -> (w255:refnum<visa-resource-name>)
            n103 = local write "stage-error"(w217) -> ()
            n104 = Unbundle By Name(w217) -> ("status"=w216:bool)
            n105 = local write "stage-stat"(w216) -> ()
            n106 = Concatenate Strings("\n\n\n\nSaving Data\nLogging started at\n" ("String"), w228) -> (w231:string)
            n107 = Unbundle By Name(w215) -> ("Bar X"=w214:dbl, "Bar Y"=w213:dbl, "PD X"=w212:dbl, "PD Y"=w211:dbl, "BMA"=w210:dbl, "PDA"=w209:dbl)
            n108 = call "meter_buffered.vi"("Samples"="nSamples", "error in"=w254, "PD ranges"=w233, "meter-VISA"=w255) -> ("error out"=w234:errorcluster, "ch1-3 data"=w242:dbl[][])  [unwired: 3 in, 3 out]
            n109 = local write "meter-error"(w234) -> ()
            n110 = Unbundle By Name(w234) -> ("status"=w235:bool)
            n111 = local write "start-msg"(w231) -> ()
            n112 = Initialize Array("bar-note", "nSamples") -> (w240:u16[])
            n113 = local write "meter-stat"(w235) -> ()
            n114 = Initialize Array(w214, "nSamples") -> (w225:dbl[])
            n115 = Initialize Array(w213, "nSamples") -> (w224:dbl[])
            n116 = Initialize Array(w212, "nSamples") -> (w223:dbl[])
            n117 = Initialize Array(w211, "nSamples") -> (w222:dbl[])
            n118 = Initialize Array(w210, "nSamples") -> (w221:dbl[])
            n119 = Initialize Array(w209, "nSamples") -> (w220:dbl[])
            n120 = Insert Into Array(array=w242, index (col)=3 ("disabled index (col)"), new element #1=w240, new element #2=w225, new element #3=w224, new element #4=w223, new element #5=w222, new element #6=w221, new element #7=w220) -> (w227:dbl[][])  [unwired: 1 in]
            n121 = local read "log-error"() -> (w252:errorcluster)
            n122 = local read "log-path"() -> (w253:path)
            n123 = Array To Spreadsheet String(delimiter (Tab)=", ", array=w227, 3:"%.6e" ("format string")) -> (spreadsheet string=w237:string)
            n124 = Open/Create/Replace File(file path (use dialog)=w253, error in=w252, operation (0:open)=T6."open", access (0:read/write)=enum16{"read/write", "read-only", "write-only"}."read/write") -> (refnum out=w251:refnum<file>, error out=w247:errorcluster)  [unwired: 2 in, 1 out]
            n125 = Read from Text File(file (use dialog)=w251, error in=w247) -> (refnum out=w248:refnum<file>, text=w207:string, error out=w246:errorcluster)  [unwired: 2 in, 1 out]
            n126 = local write "keep-file"(TRUE ("keep-file")) -> ()
            n127 = Equal?(x=w205, y=w207) -> (x = y?=w206:bool)
            n128 = Select(t="T, PD1, PD2, PD3, bar note, bar x, bar y, pd x, pd y, bma, pda\n", s=w206, f=w205) -> (s? t:f=w202:string)
            n129 = Concatenate Strings(w202, w237) -> (w203:string)
            n130 = Write to Text File(file (use dialog)=w248, text=w203, error in=w246) -> (refnum out=w250:refnum<file>, error out=w249:errorcluster)  [unwired: 1 in, 1 out]
            n131 = local read "state-queue"() -> (w230:T4)
            n132 = Close File(refnum=w250, error in=w249) -> (error out=w245:errorcluster)  [unwired: 1 out]
            n133 = Unbundle By Name(w245) -> ("status"=→"file-stat":bool)
            n134 = local write "log-error"(w245) -> ()
          }
          frame "log-pd3" {
            w269 = ""
            # "New (as of 2025-08-11) data logging:\nUse meter's internal buffering capabilities to acquire N samples and save that data to the log file."
            # "DAQ for logging to data file - runs only when initiated"
            n135 = local read "stage-error"() -> (w283:errorcluster)
            n136 = local read "Current Time:"() -> (w287:string)
            n137 = property on="start-msg" class="Str"("Visible"=TRUE) -> ()  [unwired: 2 in, 2 out]
            n138 = local read "meter-error"() -> (w257:errorcluster)
            n139 = local read "meter-visa"() -> (w259:refnum<visa-resource-name>)
            n140 = local read "PD Values"() -> (w258:cluster{"PD1":dbl, "PD2":dbl, "PD3":dbl})
            n141 = call "get-stage-positions.vi"("error in (no error)"=w283, "Cluster"=w284) -> ("error out"=w282:errorcluster, "stage positions"=w281:T2)  [unwired: 8 in]
            n142 = local read "nSamples"() -> (w260:dbl)
            n143 = local write "last-save-time"(w287) -> ()
            n144 = Cluster To Array(cluster=w281) -> (array=w266:dbl[])
            n145 = Unbundle By Name(w282) -> ("status"=w285:bool)
            n146 = local write "stage-error"(w282) -> ()
            n147 = Concatenate Strings("\n\n\n\nSaving Data\nLogging started at\n" ("String"), w287) -> (w290:string)
            n148 = call "meter_buffered.vi"("Samples"=w260, "error in"=w257, "PD ranges"=w258, "meter-VISA"=w259) -> ("error out"=w261:errorcluster, "stats-out"=w256:dbl[])  [unwired: 3 in, 3 out]
            n149 = local write "stage-stat"(w285) -> ()
            n150 = local write "start-msg"(w290) -> ()
            n151 = local write "meter-error"(w261) -> ()
            n152 = Unbundle By Name(w261) -> ("status"=w292:bool)
            n153 = Number To Fractional String(number=w266) -> (F-format string=w262:string[])  [unwired: 3 in]
            n154 = local write "meter-stat"(w292) -> ()
            n155 = Number To Exponential String(number=w256) -> (E-format string=w265:string[])  [unwired: 3 in]
            n156 = Number To Decimal String(number=w267) -> (decimal integer string=w263:string)  [unwired: 1 in]
            n157 = local write "keep-file"(TRUE ("keep-file")) -> ()
            n158 = Get Date/Time In Seconds() -> (seconds since 1Jan1904=w280:timestamp)
            n159 = Format Date/Time String(time format string (%c)="%Y-%m-%d %H:%M:%S%6u", seconds (now)=w280) -> (date/time string=w276:string)  [unwired: 1 in]
            n160 = Build Array (concatenate)(w265, w263, w262) -> (w264:string[])
            n161 = local read "log-error"() -> (w304:errorcluster)
            n162 = local read "log-path"() -> (w305:path)
            n163 = Insert Into Array(array=w264, index=0, new element=w276) -> (w277:string[])
            n164 = Open/Create/Replace File(file path (use dialog)=w305, error in=w304, operation (0:open)=T6."open", access (0:read/write)=enum16{"read/write", "read-only", "write-only"}."read/write") -> (refnum out=w303:refnum<file>, error out=w299:errorcluster)  [unwired: 2 in, 1 out]
            n165 = Array To Spreadsheet String(delimiter (Tab)=", ", array=w277, 3:"%s" ("format string")) -> (spreadsheet string=w293:string)
            n166 = Read from Text File(file (use dialog)=w303, error in=w299) -> (refnum out=w300:refnum<file>, text=w273:string, error out=w298:errorcluster)  [unwired: 2 in, 1 out]
            n167 = Equal?(x=w269, y=w273) -> (x = y?=w270:bool)
            n168 = Select(t="T, PD1 avg, PD1 stdev, PD2 avg, PD2 stdev, PD3 avg, PD3 stdev, bar note, bar x, bar y, pd x, pd y, bma, pda\n", s=w270, f=w269) -> (s? t:f=w271:string)
            n169 = Concatenate Strings(w271, w293) -> (w272:string)
            n170 = Write to Text File(file (use dialog)=w300, text=w272, error in=w298) -> (refnum out=w302:refnum<file>, error out=w301:errorcluster)  [unwired: 1 in, 1 out]
            n171 = Close File(refnum=w302, error in=w301) -> (error out=w297:errorcluster)  [unwired: 1 out]
            n172 = Unbundle By Name(w297) -> ("status"=w286:bool)
            n173 = local write "log-error"(w297) -> ()
            n174 = local read "state-queue"() -> (w289:T4)
            n175 = local write "file-stat"(w286) -> ()
          }
          frame "move" {
            w306 = 12000 ("waitTimeout")
            # "Move stages to pre-defined positions - runs only when initiated"
            n176 = Unbundle By Name(w327) -> ("PDX"=w326:dbl, "PDY"=w325:dbl, "BarX"=w324:dbl, "BarY"=w323:dbl, "BMA"=w322:dbl, "PDA"=w321:dbl)  [unwired: 1 out]
            n177 = local read "bar-note"() -> (w332:u16)
            n178 = property on="start-msg" class="Str"("Visible"=TRUE) -> ()  [unwired: 2 in, 2 out]
            n179 = local write "start-msg"("\n\n\nMOVING\nSTAGES\n\nPlease wait..." ("String")) -> ()
            n180 = local write "BarY"(w323) -> ()
            n181 = local write "BMA"(w322) -> ()
            n182 = local write "PDX"(w326) -> ()
            n183 = local write "PDY"(w325) -> ()
            n184 = local write "BarX"(w324) -> ()
            n185 = local write "PDA"(w321) -> ()
            n186 = local write "bar-note"(w332) -> ()
            n187 = Unbundle By Name(w331) -> ("PD X"=w312:refnum<k24>, "PD Y"=w307:refnum<k24>, "Bar X"=w308:refnum<k24>, "Bar Y"=w309:refnum<k24>, "Brewster"=w310:refnum<k24>, "PD Angle"=w311:refnum<k24>)
            n188 = invoke class="IntegratedStepperMotor" method="MoveTo"(reference=w312, "position"=w326, "waitTimeout"=w306) -> (error out=w319:errorcluster)  [unwired: 2 in, 4 out]
            n189 = invoke class="IntegratedStepperMotor" method="MoveTo"(reference=w307, "position"=w325, "waitTimeout"=w306) -> (error out=w318:errorcluster)  [unwired: 2 in, 4 out]
            n190 = invoke class="StepperMotorChannel" method="MoveTo"(reference=w310, "position"=w322, "waitTimeout"=w306) -> (error out=w315:errorcluster)  [unwired: 2 in, 4 out]
            n191 = invoke class="StepperMotorChannel" method="MoveTo"(reference=w311, "position"=w321, "waitTimeout"=w306) -> (error out=w314:errorcluster)  [unwired: 2 in, 4 out]
            n192 = invoke class="IntegratedStepperMotor" method="MoveTo"(reference=w308, "position"=w324, "waitTimeout"=w306) -> (error out=w317:errorcluster)  [unwired: 2 in, 4 out]
            n193 = invoke class="IntegratedStepperMotor" method="MoveTo"(reference=w309, "position"=w323, "waitTimeout"=w306) -> (error out=w316:errorcluster)  [unwired: 2 in, 4 out]
            n194 = local read "stage-error"() -> (w320:errorcluster)
            n195 = Merge Errors(w320, w319, w318, w317, w316, w315, w314) -> (w313:errorcluster)
            n196 = local write "stage-error"(w313) -> ()
            n197 = local read "state-queue"() -> (w330:T4)
          }
          frame "diode-scan" {
            # "PDX  262-268\nPDY 120.5 -126.5\nLaser 45\nPD   180.5"
            n198 = local read "state-queue"() -> (w343:T4)
            n199 = call "build-diode-scan-pts.vi"("Y step size"="Y step size", "X step size"="X step size", "Y end"="Y end", "Y start"="Y start", "X end"="X end", "X start"="X start") -> ("y"=w341:dbl[], "x"=w342:dbl[])  [unwired: 4 in]
            n200 = for {
              tunnel: w342 -> [w357] mode=indexing
              tunnel: w341 -> [w356] mode=indexing
              shift-right: [w350] -> w340
              shift-left: w343 -> [w352]
              n201 = local read "next-state-cluster-const"() -> (w344:T1)
              n202 = Bundle By Name(cluster=w344, "next-state"="move", "bypass-confirm"=TRUE, "PDX"=w357, "PDY"=w356, "BarX"=93.0, "BarY"=20.0, "BMA"=45.0, "PDA"=180.5) -> (w351:T1)
              n203 = Bundle By Name(cluster=w344, "next-state"="log-pd3") -> (w345:T1)
              n204 = Build Array (concatenate)(w352, w351, w345) -> (w350:T4)
            }
            n205 = Array Size(array=w340) -> (size(s)=→"queue-size":i32)
          }
          frame "diode-scan-center" {
            w361 = 2.0 ("y")
            w360 = 2.0 ("y")
            # "PDX  262-268\nPDY 120.5 -126.5\nLaser 45\nPD   180.5"
            n206 = local read "stage-error"() -> (w369:errorcluster)
            n207 = call "get-stage-positions.vi"("error in (no error)"=w369, "Cluster"=w366) -> ("error out"=w368:errorcluster, "stage positions"=w367:T2)  [unwired: 8 in]
            n208 = Unbundle By Name(w368) -> ("status"=w370:bool)
            n209 = local write "stage-error"(w368) -> ()
            n210 = local write "stage-stat"(w370) -> ()
            n211 = Unbundle By Name(w367) -> ("PD X"=w365:dbl, "PD Y"=w362:dbl)
            n212 = Subtract(x=w365, y=w360) -> (x-y=w364:dbl)
            n213 = Subtract(x=w362, y=w361) -> (x-y=w359:dbl)
            n214 = Add(x=w365, y=w360) -> (x+y=w363:dbl)
            n215 = Add(x=w362, y=w361) -> (x+y=w358:dbl)
            n216 = local read "Y step size"() -> (w372:dbl)
            n217 = local read "X step size"() -> (w373:dbl)
            n218 = local read "state-queue"() -> (w377:T4)
            n219 = call "build-diode-scan-pts.vi"("Y step size"=w372, "X step size"=w373, "Y end"=w358, "Y start"=w359, "X end"=w363, "X start"=w364) -> ("y"=w375:dbl[], "x"=w376:dbl[])  [unwired: 4 in]
            n220 = for {
              tunnel: w376 -> [w391] mode=indexing
              tunnel: w375 -> [w390] mode=indexing
              shift-right: [w384] -> w374
              shift-left: w377 -> [w386]
              n221 = local read "next-state-cluster-const"() -> (w378:T1)
              n222 = Bundle By Name(cluster=w378, "next-state"="move", "bypass-confirm"=TRUE, "PDX"=w391, "PDY"=w390, "BarX"=93.0, "BarY"=20.0, "BMA"=45.0, "PDA"=181.0) -> (w385:T1)
              n223 = Bundle By Name(cluster=w378, "next-state"="log-pd3") -> (w379:T1)
              n224 = Build Array (concatenate)(w386, w385, w379) -> (w384:T4)
            }
            n225 = Array Size(array=w374) -> (size(s)=w371:i32)
            n226 = local write "queue-size"(w371) -> ()
          }
          frame "wait" {
            n227 = property on="start-msg" class="Str"("Visible"=TRUE) -> ()  [unwired: 2 in, 2 out]
            n228 = local write "start-msg"("\n\n\nProgram Delay Active\nfor User to Exit Laser Area" ("String")) -> ()
            n229 = Unbundle By Name(w395) -> ("PDX"=w396:dbl)
            n230 = Multiply(x=w396, y=1000.0) -> (x*y=w398:dbl)
            n231 = Wait (ms)(milliseconds to wait=w398) -> ()  [unwired: 1 out]
            n232 = local read "state-queue"() -> (w394:T4)
          }
          frame "align-setup" {
            n233 = Unbundle By Name(w405) -> ("bypass-confirm"=w401:bool)
            n234 = Select(t="gr-asc", s=w401, f="nelder-mead") -> (s? t:f=w404:string)
            n235 = case shown="False" "align-only" {
              tunnel: w404 -> [w411 w417]
              tunnel: [w406 w420] -> w400
              frame False {
                n236 = local read "Test Start Delay (s)"() -> (w413:dbl)
                n237 = local read "next-state-cluster-const"() -> (w407:T1)
                n238 = local read "state-queue"() -> (w415:T4)
                n239 = Bundle By Name(cluster=w407, "next-state"="wait", "PDX"=w413) -> (w412:T1)
                n240 = Bundle By Name(cluster=w407, "next-state"=w411) -> (w409:T1)
                n241 = Bundle By Name(cluster=w407, "next-state"="diode-scan-center") -> (w408:T1)
                n242 = Build Array (concatenate)(w415, w412, w409, w408) -> (w406:T4)
              }
              frame True {
                n243 = local read "next-state-cluster-const"() -> (w416:T1)
                n244 = Bundle By Name(cluster=w416, "next-state"=w417) -> (w418:T1)
                n245 = local read "state-queue"() -> (w419:T4)
                n246 = Build Array (concatenate)(w419, w418) -> (w420:T4)
              }
            }
          }
          frame "nelder-mead" {
            w426 = ""
            n247 = property on="start-msg" class="Str"("Visible"=TRUE) -> ()  [unwired: 2 in, 2 out]
            n248 = local read "stage-error"() -> (w457:errorcluster)
            n249 = call "get-stage-positions.vi"("error in (no error)"=w457, "Cluster"=w442) -> ("error out"=w456:errorcluster, "stage positions"=w455:T2)  [unwired: 8 in]
            n250 = Unbundle By Name(w456) -> ("status"=w458:bool)
            n251 = local write "stage-error"(w456) -> ()
            n252 = local write "stage-stat"(w458) -> ()
            n253 = local read "meter-error"() -> (w462:errorcluster)
            n254 = local read "stage-error"() -> (w461:errorcluster)
            n255 = local read "meter-visa"() -> (w460:refnum<visa-resource-name>)
            n256 = local read "PD Values"() -> (w459:cluster{"PD1":dbl, "PD2":dbl, "PD3":dbl})
            n257 = local write "start-msg"("\n\n\n\nPerforming Automated\nAlignment.\n\nPlease Wait.\n" ("String")) -> ()
            n258 = Unbundle By Name(w455) -> ("PD Y"=w453:dbl, "PD X"=w454:dbl)
            n259 = Bundle By Name(cluster=T7 {"alpha"=1.0, "gamma"=2.0, "rho"=0.5, "sigma"=0.5, "simplex L"=0.5} ("NM-params"), "simplex L"=0.5, "sigma"=0.5) -> (w445:T7)
            n260 = call "auto_alignment-v3-1.vi"("meter-visa"=w460, "xStart"=w454, "yStart"=w453, "NM-params"=w445, "PD Values"=w459, "stage-refs"=w442, "meter-error"=w462, "stage-error"=w461, "bar-note"=w441, "meas#"=w440) -> ("Optimized Location"=→"Optimized Location":dbl[], "logfile-line-out"=w423:string, "meter-error-out"=w452:errorcluster, "run time (s)"=→"run time (min)":dbl, "stage-error-out"=w451:errorcluster)  [unwired: 1 in]
            n261 = local write "meter-error"(w452) -> ()
            n262 = local write "stage-error"(w451) -> ()
            n263 = local write "keep-file"(TRUE ("keep-file")) -> ()
            n264 = local read "log-error"() -> (w438:errorcluster)
            n265 = local read "log-path"() -> (w439:path)
            n266 = Open/Create/Replace File(file path (use dialog)=w439, error in=w438, operation (0:open)=T6."open", access (0:read/write)=enum16{"read/write", "read-only", "write-only"}."read/write") -> (refnum out=w437:refnum<file>, error out=w433:errorcluster)  [unwired: 2 in, 1 out]
            n267 = Read from Text File(file (use dialog)=w437, error in=w433) -> (refnum out=w434:refnum<file>, text=w430:string, error out=w432:errorcluster)  [unwired: 2 in, 1 out]
            n268 = Equal?(x=w426, y=w430) -> (x = y?=w429:bool)
            n269 = Select(t="time\tpd1\tpd2\tpd3\tpd3/pd1\tpd2/pd1\tbx\tby\tpdx\tpdy\tpda\tbm\tbar-note\tmeas#\tpt#\n", s=w429, f=w426) -> (s? t:f=w427:string)
            n270 = Concatenate Strings(w427, w423) -> (w428:string)
            n271 = Write to Text File(file (use dialog)=w434, text=w428, error in=w432) -> (refnum out=w436:refnum<file>, error out=w435:errorcluster)  [unwired: 1 in, 1 out]
            n272 = Close File(refnum=w436, error in=w435) -> (error out=w431:errorcluster)  [unwired: 1 out]
            n273 = Unbundle By Name(w431) -> ()  [unwired: 1 out]
            n274 = local write "log-error"(w431) -> ()
            n275 = local read "state-queue"() -> (w463:T4)
          }
          frame "multi-trial" {
            n276 = local read "next-state-cluster-const"() -> (w464:T1)
            n277 = Initialize Array(w464, 0 ("dimension size")) -> (w472:T4)
            n278 = for {
              N: 20 -> [_]
              shift-right: [w493] -> w467
              shift-left: w472 -> [w494]
              tunnel: "PDX start" -> [w481]
              tunnel: "PDY start" -> [w477]
              w476 = 2.0
              n279 = Subtract(x=w477, y=w476) -> (x-y=w478:dbl)
              n280 = local read "bar-note"() -> (w474:u16)
              n281 = Add(x=w477, y=w476) -> (x+y=w479:dbl)
              n282 = Subtract(x=w481, y=w476) -> (x-y=w483:dbl)
              n283 = Add(x=w481, y=w476) -> (x+y=w482:dbl)
              n284 = call-poly <vilib>:"Random Number (Range).vi"("lower bound (0)"=w478, "upper bound (100)"=w479) -> ("number"=w475:dbl)  [unwired: 9 in]
              n285 = call-poly <vilib>:"Random Number (Range).vi"("lower bound (0)"=w483, "upper bound (100)"=w482) -> ("number"=w480:dbl)  [unwired: 9 in]
              n286 = local read "next-state-cluster-const"() -> (w490:T1)
              n287 = Bundle By Name(cluster=w490, "next-state"="move", "bypass-confirm"=TRUE, "PDX"=w480, "PDY"=w475, "BarX"=90.0, "BarY"=35.0, "BMA"=45.0, "PDA"=181.0, "bar-note"=w474) -> (w491:T1)
              n288 = Bundle By Name(cluster=w490, "next-state"="nelder-mead") -> (w492:T1)
              n289 = Build Array (concatenate)(w494, w491, w492) -> (w493:T4)
            }
            n290 = Bundle By Name(cluster=w464, "next-state"="diode-scan-center") -> (w465:T1)
            n291 = Build Array (concatenate)(w467, w465) -> (w466:T4)
          }
          frame "setup-IR" {
            # "Pure Beam (PB)\nPDX 266\nPDY 126\nBX 170\nBY 30\nBA 45\nPDA 180"
            # "IR1\nPDX 232\nPDY 119.5\nBX 85\nBY 20\nBA 17.148\nPDA 238\n\nIR2\nPDX 232\nPDY 119.5\nBX 85\nBY 15\nBA 17.148\nPDA 238\n\nIR3\nPDX 232\nPDY 119.5\nBX 85\nBY 32\nBA 17.148\nPDA 238"
            n292 = local read "state-queue"() -> (w505:T4)
            n293 = for {
              N: 10 -> [_]
              shift-right: [w605] -> w501
              shift-left: w505 -> [w613]
              shift-right: [w589] -> w502
              shift-left: u32 0 -> [w586]
              i -> [w604]
              # "PB"
              # "IR1"
              n294 = Multiply(x=0.1, y=w604) -> (x*y=w596:dbl)
              n295 = local read "next-state-cluster-const"() -> (w592:T1)
              n296 = Add(x=20.0, y=w596) -> (x+y=w582:dbl)
              n297 = Add(x=85.0, y=w596) -> (x+y=w583:dbl)
              n298 = Add(x=30.0, y=w596) -> (x+y=w579:dbl)
              n299 = Add(x=170.0, y=w596) -> (x+y=w578:dbl)
              n300 = Bundle By Name(cluster=w592, "next-state"="move", "bypass-confirm"=TRUE, "PDX"=223.0 ("BarX"), "PDY"=119.5 ("BarY"), "BarX"=w583, "BarY"=w582, "BMA"=17.148, "PDA"=238.0) -> (w609:T1)
              n301 = Bundle By Name(cluster=w592, "next-state"="move", "bypass-confirm"=TRUE, "PDX"=266.0 ("BarX"), "PDY"=126.0 ("BarY"), "BarX"=w578, "BarY"=w579, "BMA"=45.0, "PDA"=180.0) -> (w591:T1)
              n302 = Increment(x=w586) -> (x+1=w589:u32)
              n303 = Bundle By Name(cluster=w592, "next-state"="nelder-mead", "bar-note"=u8 1, "meas#"=w586) -> (w606:T1)
              n304 = Bundle By Name(cluster=w592, "next-state"="nelder-mead", "bar-note"=u8 0, "meas#"=w586) -> (w590:T1)
              n305 = Build Array (concatenate)(w613, w609, w606, w591, w590) -> (w605:T4)
            }
            n306 = for {
              N: 10 -> [_]
              shift-right: [w569] -> w499
              shift-left: w501 -> [w577]
              shift-right: [w553] -> w498
              shift-left: w502 -> [w550]
              i -> [w568]
              # "PB"
              # "IR1"
              n307 = Multiply(x=0.1, y=w568) -> (x*y=w560:dbl)
              n308 = local read "next-state-cluster-const"() -> (w556:T1)
              n309 = Add(x=20.0, y=w560) -> (x+y=w546:dbl)
              n310 = Add(x=85.0, y=w560) -> (x+y=w547:dbl)
              n311 = Add(x=30.0, y=w560) -> (x+y=w543:dbl)
              n312 = Add(x=170.0, y=w560) -> (x+y=w542:dbl)
              n313 = Bundle By Name(cluster=w556, "next-state"="move", "bypass-confirm"=TRUE, "PDX"=223.0 ("BarX"), "PDY"=119.5 ("BarY"), "BarX"=w547, "BarY"=w546, "BMA"=17.148, "PDA"=238.0) -> (w573:T1)
              n314 = Bundle By Name(cluster=w556, "next-state"="move", "bypass-confirm"=TRUE, "PDX"=266.0 ("BarX"), "PDY"=126.0 ("BarY"), "BarX"=w542, "BarY"=w543, "BMA"=45.0, "PDA"=180.0) -> (w555:T1)
              n315 = Increment(x=w550) -> (x+1=w553:u32)
              n316 = Bundle By Name(cluster=w556, "next-state"="nelder-mead", "bar-note"=u8 1, "meas#"=w550) -> (w570:T1)
              n317 = Bundle By Name(cluster=w556, "next-state"="nelder-mead", "bar-note"=u8 0, "meas#"=w550) -> (w554:T1)
              n318 = Build Array (concatenate)(w577, w573, w570, w555, w554) -> (w569:T4)
            }
            n319 = for {
              N: 10 -> [_]
              shift-right: [w533] -> w496
              shift-left: w499 -> [w541]
              shift-right: [w517] -> _
              shift-left: w498 -> [w514]
              i -> [w532]
              # "PB"
              # "IR1"
              n320 = Multiply(x=0.1, y=w532) -> (x*y=w524:dbl)
              n321 = local read "next-state-cluster-const"() -> (w520:T1)
              n322 = Add(x=20.0, y=w524) -> (x+y=w510:dbl)
              n323 = Add(x=85.0, y=w524) -> (x+y=w511:dbl)
              n324 = Add(x=30.0, y=w524) -> (x+y=w507:dbl)
              n325 = Add(x=170.0, y=w524) -> (x+y=w506:dbl)
              n326 = Bundle By Name(cluster=w520, "next-state"="move", "bypass-confirm"=TRUE, "PDX"=223.0 ("BarX"), "PDY"=119.5 ("BarY"), "BarX"=w511, "BarY"=w510, "BMA"=17.148, "PDA"=238.0) -> (w537:T1)
              n327 = Bundle By Name(cluster=w520, "next-state"="move", "bypass-confirm"=TRUE, "PDX"=266.0 ("BarX"), "PDY"=126.0 ("BarY"), "BarX"=w506, "BarY"=w507, "BMA"=45.0, "PDA"=180.0) -> (w519:T1)
              n328 = Increment(x=w514) -> (x+1=w517:u32)
              n329 = Bundle By Name(cluster=w520, "next-state"="nelder-mead", "bar-note"=u8 1, "meas#"=w514) -> (w534:T1)
              n330 = Bundle By Name(cluster=w520, "next-state"="nelder-mead", "bar-note"=u8 0, "meas#"=w514) -> (w518:T1)
              n331 = Build Array (concatenate)(w541, w537, w534, w519, w518) -> (w533:T4)
            }
          }
          frame "setup-BA" {
            # "Pure Beam (PB)\nPDX 266\nPDY 126\nBX 170\nBY 30\nBA 45\nPDA 180"
            # "BA1\nPDX 268\nPDY 126\nBX 229\nBY 30\nBA 45\nPDA 180\n\nBA2\nPDX 268\nPDY 126\nBX 229\nBY 15\nBA 45\nPDA 180\n\nBA3\nPDX 268\nPDY 126\nBX 229\nBY 20\nBA 45\nPDA 180"
            n332 = local read "state-queue"() -> (w623:T4)
            n333 = for {
              N: 10 -> [_]
              shift-right: [w723] -> w620
              shift-left: w623 -> [w731]
              shift-right: [w707] -> w618
              shift-left: u32 0 -> [w704]
              i -> [w722]
              # "PB"
              # "BA1"
              n334 = Multiply(x=0.1, y=w722) -> (x*y=w714:dbl)
              n335 = local read "next-state-cluster-const"() -> (w710:T1)
              n336 = Add(x=30.0, y=w714) -> (x+y=w700:dbl)
              n337 = Add(x=30.0, y=w714) -> (x+y=w696:dbl)
              n338 = Add(x=229.0, y=w714) -> (x+y=w701:dbl)
              n339 = Add(x=170.0, y=w714) -> (x+y=w697:dbl)
              n340 = Bundle By Name(cluster=w710, "next-state"="move", "bypass-confirm"=TRUE, "PDX"=268.0 ("BarX"), "PDY"=126.0 ("BarY"), "BarX"=w701, "BarY"=w700, "BMA"=45.0, "PDA"=180.0) -> (w727:T1)
              n341 = Bundle By Name(cluster=w710, "next-state"="move", "bypass-confirm"=TRUE, "PDX"=266.0 ("BarX"), "PDY"=126.0 ("BarY"), "BarX"=w697, "BarY"=w696, "BMA"=45.0, "PDA"=180.0) -> (w709:T1)
              n342 = Increment(x=w704) -> (x+1=w707:u32)
              n343 = Bundle By Name(cluster=w710, "next-state"="nelder-mead", "bar-note"=u8 2, "meas#"=w704) -> (w724:T1)
              n344 = Bundle By Name(cluster=w710, "next-state"="nelder-mead", "bar-note"=u8 0, "meas#"=w704) -> (w708:T1)
              n345 = Build Array (concatenate)(w731, w727, w724, w709, w708) -> (w723:T4)
            }
            n346 = for {
              N: 10 -> [_]
              shift-right: [w651] -> w619
              shift-left: w620 -> [w659]
              shift-right: [w635] -> w617
              shift-left: w618 -> [w632]
              i -> [w650]
              # "PB"
              # "BA2"
              n347 = Multiply(x=0.1, y=w650) -> (x*y=w642:dbl)
              n348 = local read "next-state-cluster-const"() -> (w638:T1)
              n349 = Add(x=15.0, y=w642) -> (x+y=w628:dbl)
              n350 = Add(x=30.0, y=w642) -> (x+y=w624:dbl)
              n351 = Add(x=229.0, y=w642) -> (x+y=w629:dbl)
              n352 = Add(x=170.0, y=w642) -> (x+y=w625:dbl)
              n353 = Bundle By Name(cluster=w638, "next-state"="move", "bypass-confirm"=TRUE, "PDX"=268.0 ("BarX"), "PDY"=126.0 ("BarY"), "BarX"=w629, "BarY"=w628, "BMA"=45.0, "PDA"=180.0) -> (w655:T1)
              n354 = Bundle By Name(cluster=w638, "next-state"="move", "bypass-confirm"=TRUE, "PDX"=266.0 ("BarX"), "PDY"=126.0 ("BarY"), "BarX"=w625, "BarY"=w624, "BMA"=45.0, "PDA"=180.0) -> (w637:T1)
              n355 = Increment(x=w632) -> (x+1=w635:u32)
              n356 = Bundle By Name(cluster=w638, "next-state"="nelder-mead", "bar-note"=u8 2, "meas#"=w632) -> (w652:T1)
              n357 = Bundle By Name(cluster=w638, "next-state"="nelder-mead", "bar-note"=u8 0, "meas#"=w632) -> (w636:T1)
              n358 = Build Array (concatenate)(w659, w655, w652, w637, w636) -> (w651:T4)
            }
            n359 = for {
              N: 10 -> [_]
              shift-right: [w687] -> w614
              shift-left: w619 -> [w695]
              shift-right: [w671] -> _
              shift-left: w617 -> [w668]
              i -> [w686]
              # "PB"
              # "BA3"
              n360 = Multiply(x=0.1, y=w686) -> (x*y=w678:dbl)
              n361 = local read "next-state-cluster-const"() -> (w674:T1)
              n362 = Add(x=20.0, y=w678) -> (x+y=w664:dbl)
              n363 = Add(x=30.0, y=w678) -> (x+y=w660:dbl)
              n364 = Add(x=229.0, y=w678) -> (x+y=w665:dbl)
              n365 = Add(x=170.0, y=w678) -> (x+y=w661:dbl)
              n366 = Bundle By Name(cluster=w674, "next-state"="move", "bypass-confirm"=TRUE, "PDX"=268.0 ("BarX"), "PDY"=126.0 ("BarY"), "BarX"=w665, "BarY"=w664, "BMA"=45.0, "PDA"=180.0) -> (w691:T1)
              n367 = Bundle By Name(cluster=w674, "next-state"="move", "bypass-confirm"=TRUE, "PDX"=266.0 ("BarX"), "PDY"=126.0 ("BarY"), "BarX"=w661, "BarY"=w660, "BMA"=45.0, "PDA"=180.0) -> (w673:T1)
              n368 = Increment(x=w668) -> (x+1=w671:u32)
              n369 = Bundle By Name(cluster=w674, "next-state"="nelder-mead", "bar-note"=u8 2, "meas#"=w668) -> (w688:T1)
              n370 = Bundle By Name(cluster=w674, "next-state"="nelder-mead", "bar-note"=u8 0, "meas#"=w668) -> (w672:T1)
              n371 = Build Array (concatenate)(w695, w691, w688, w673, w672) -> (w687:T4)
            }
          }
        }
        n372 = Subtract(x=w106, y=w105) -> (x-y=→"loop-rate":u32)
        n373 = Get Date/Time In Seconds() -> (seconds since 1Jan1904=w101:timestamp)
        n374 = Format Date/Time String(time format string (%c)="%Y-%m-%d %H:%M:%S", seconds (now)=w101) -> (date/time string=→"Current Time:":string)  [unwired: 1 in]
      }
    }
    frame #4 {
      # "close stages"
      n375 = local read "main-stage-refs"() -> (w732:T3)
      n376 = Unbundle By Name(w732) -> ("Bar X main"=w738:refnum<k24>, "Bar Y main"=w737:refnum<k24>, "PD X main"=w736:refnum<k24>, "PD Y main"=w735:refnum<k24>, "BMA main"=w734:refnum<k24>, "PDA main"=w733:refnum<k24>)
      n377 = invoke class="BenchtopStepperControl" method="CloseDevice"(reference=w734) -> (error out=w743:errorcluster)  [unwired: 2 in, 2 out]
      n378 = invoke class="BenchtopStepperControl" method="CloseDevice"(reference=w733) -> (error out=w744:errorcluster)  [unwired: 2 in, 2 out]
      n379 = invoke class="LongTravelStageControl" method="CloseDevice"(reference=w738) -> (error out=w739:errorcluster)  [unwired: 2 in, 2 out]
      n380 = invoke class="LongTravelStageControl" method="CloseDevice"(reference=w737) -> (error out=w740:errorcluster)  [unwired: 2 in, 2 out]
      n381 = invoke class="LongTravelStageControl" method="CloseDevice"(reference=w736) -> (error out=w741:errorcluster)  [unwired: 2 in, 2 out]
      n382 = invoke class="LongTravelStageControl" method="CloseDevice"(reference=w735) -> (error out=w742:errorcluster)  [unwired: 2 in, 2 out]
      n383 = local read "stage-error"() -> (w745:errorcluster)
      n384 = Merge Errors(w745, w739, w740, w741, w742, w743, w744) -> (w746:errorcluster)
      n385 = local write "stage-error"(w746) -> ()
    }
    frame #5 {
      # "Close connection to meter"
      n386 = local read "meter-error"() -> (w748:errorcluster)
      n387 = local read "meter-visa"() -> (w747:refnum<visa-resource-name>)
      n388 = call <instrlib>:"Close.vi"("error in (no error)"=w748, "VISA resource name"=w747) -> ("error out"=w749:errorcluster)  [unwired: 9 in]
      n389 = local write "meter-error"(w749) -> ()
    }
    frame #6 {
      # "Section deletes log file if nothing is written to it\nto prevent just a ton of empty files during development"
      n390 = local read "log-error"() -> (w752:errorcluster)
      n391 = local read "keep-file"() -> (w750:bool)
      n392 = local read "log-path"() -> (w751:path)
      n393 = case shown="False" w750 {
        tunnel: w752 -> [w755 w757]
        tunnel: [w756 w757] -> w753
        tunnel: w751 -> [w754 _]
        frame False {
          n394 = Delete(path (use dialog)=w754, error in=w755) -> (error out=w756:errorcluster)  [unwired: 3 in, 2 out]
        }
        frame True {
        }
      }
      n395 = local write "log-error"(w753) -> ()
    }
  }
